vi "test_F9P_ubx-check-2.vi"() -> ()   [LabVIEW 2019]
uses:
  Ctrl/gnss_config.ctl
  Ctrl/ubx-packet.ctl
panel:
  in  "add str":bool=TRUE
  out "ubx arr":T1[](array[typedef])
  in  "GNSS cfg":T2={"Port"="COM10", "heading select"="", "PwrPak7_mode select"=[], "rate"=115200}
  out "buff-n":u32(graph)
  out "data check":bool
  out "error out":errorcluster
  out "n":i32
  out "GNGGA_val":bool
  out "LatLong":cluster{dbl, dbl} {"?" format="%.11f"; "?" format="%.12f"}
  in  "graph arr":bool
  out "XY 그래프":cluster{"X":dbl, "Y":dbl}[](graph)
  in  "정지":bool
  out "연결된 문자열":string
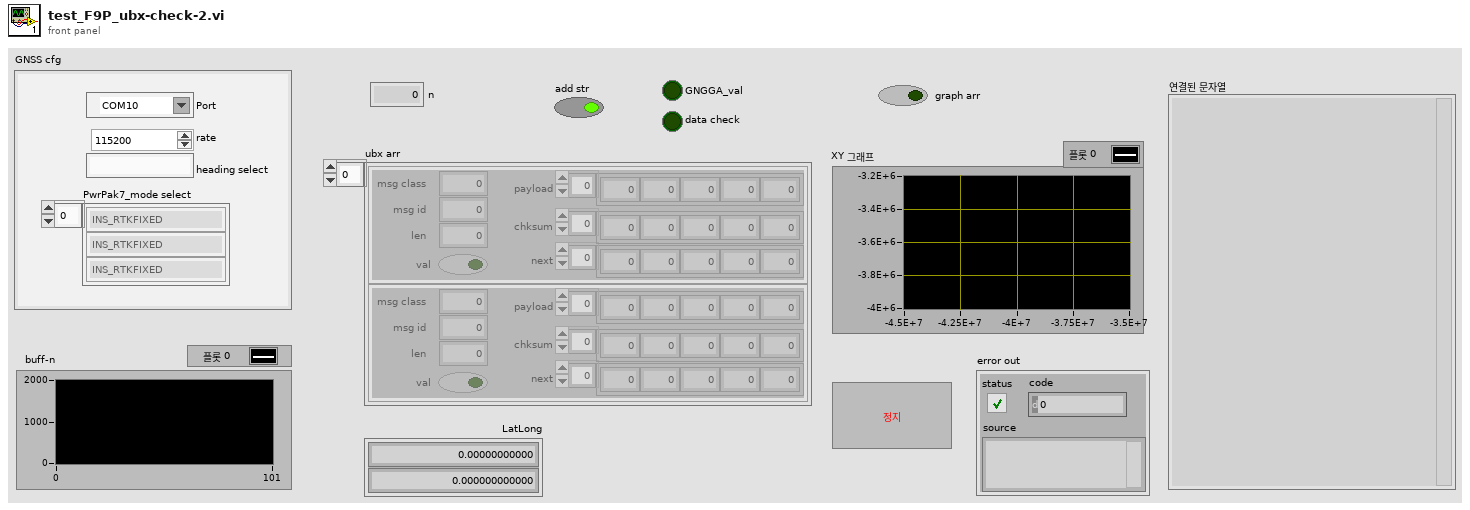
[diagram p1: front panel]
types:
  T1 = typedef "ubx-packet.ctl" = cluster{"msg class":u8, "msg id":u8, "len":u8, "payload":u8[], "chksum":u8[], "next ":u8[], "val":bool}
  T2 = typedef "gnss_config.ctl" = cluster{"Port":refnum<visa-resource-name>, "heading select":string, "PwrPak7_mode select":string[], "rate":u32}
  T3 = enum16{"GxDTM", "GxGBS", "GxGGA", "GxGLL", "GxGNS", "GxGRS", "GxGSA", "GxGST", "GxGSV", "GxRLM", "GxRMC", "GxTHS", "GxTXT", "GxVLW", "GxVTG", "GxZDA"}
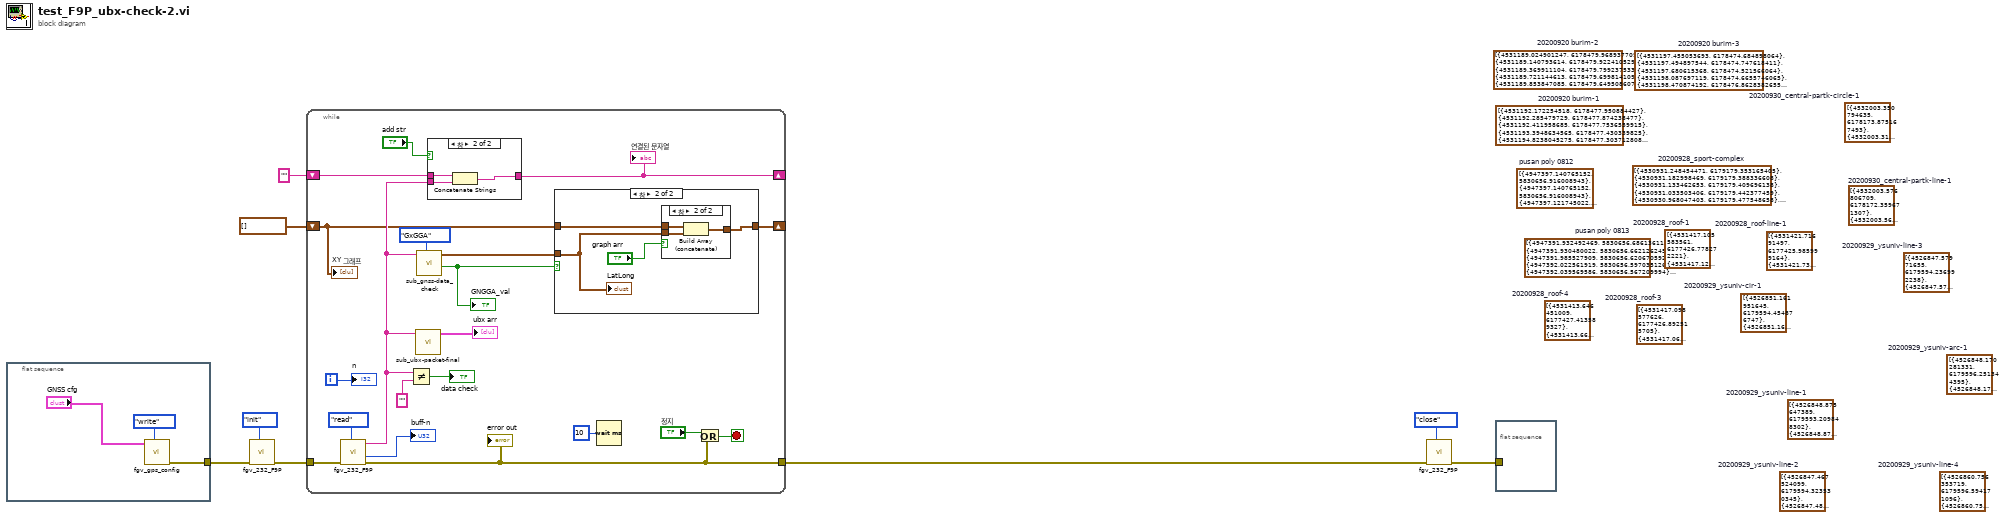
[diagram p0: block diagram]
diagram:
  (unwired) cluster{"X":dbl, "Y":dbl}[] [{"X"=4532003.350794635, "Y"=6178173.875167493}, {"X"=4532003.318056276, "Y"=6178173.892770662}, {"X"=4532003.1579189105, "Y"=6178174.020957441}, {"X"=4532002.967709019, "Y"=6178174.196875582}, {"X"=4532002.672245268, "Y"=6178174.539853451}, {"X"=4532002.3370043775, "Y"=6178175.014684652}, {"X"=4532002.006206528, "Y"=6178175.539729376}, {"X"=4532001.675408691, "Y"=6178176.064773935}, {"X"=4532001.257877701, "Y"=6178176.578591164}, {"X"=4532000.912932229, "Y"=6178177.1375437835}, {"X"=4532000.552950506, "Y"=6178177.72036187}, {"X"=4532000.193857393, "Y"=6178178.313222488}, {"X"=4531999.835652887, "Y"=6178178.916125633}, {"X"=4531999.476559786, "Y"=6178179.508985873}, {"X"=4531998.959036802, "Y"=6178180.055525806}, {"X"=4531998.308713558, "Y"=6178180.457800657}, {"X"=4531997.609657364, "Y"=6178180.696909645}, {"X"=4531996.896383714, "Y"=6178180.775335258}, {"X"=4531996.09371134, "Y"=6178180.812405522}, {"X"=4531995.219342304, "Y"=6178180.814383002}, {"X"=4531994.477703708, "Y"=6178180.766033763}, {"X"=4531993.713031512, "Y"=6178180.651165896}, {"X"=4531992.935100371, "Y"=6178180.580249076}, {"X"=4531992.061620369, "Y"=6178180.592269521}, {"X"=4531991.173992895, "Y"=6178180.638198248}, {"X"=4531990.289920003, "Y"=6178180.724297736}, {"X"=4531989.372220418, "Y"=6178180.817957572}, {"X"=4531988.393487616, "Y"=6178180.997036841}, {"X"=4531987.627109124, "Y"=6178181.056675129}, {"X"=4531986.969538497, "Y"=6178180.989425519}, {"X"=4531986.427884561, "Y"=6178180.875629432}, {"X"=4531985.817199784, "Y"=6178180.75686876}, {"X"=4531985.116227672, "Y"=6178180.586710377}, {"X"=4531984.448882404, "Y"=6178180.408991751}, {"X"=4531983.6541389, "Y"=6178180.341855931}, {"X"=4531982.97797792, "Y"=6178180.258301622}, {"X"=4531982.517725303, "Y"=6178180.095477112}, {"X"=4531982.130876179, "Y"=6178179.793239902}, {"X"=4531982.0643702205, "Y"=6178179.429221983}, {"X"=4531982.268655881, "Y"=6178179.024806436}, {"X"=4531982.716326828, "Y"=6178178.6578521365}, {"X"=4531983.194958756, "Y"=6178178.253209357}, {"X"=4531983.691292785, "Y"=6178177.854828909}, {"X"=4531984.013272379, "Y"=6178177.4239516035}, {"X"=4531984.440575617, "Y"=6178177.020606336}, {"X"=4531984.7652211515, "Y"=6178176.619856802}, {"X"=4531985.021724419, "Y"=6178176.224185293}, {"X"=4531985.4543595435, "Y"=6178175.881095707}, {"X"=4531985.720637784, "Y"=6178175.595893426}, {"X"=4531986.162159305, "Y"=6178175.353230416}, {"X"=4531986.617828416, "Y"=6178175.076659101}, {"X"=4531987.01861415, "Y"=6178174.761214936}, {"X"=4531987.26185866, "Y"=6178174.409493832}, {"X"=4531987.470587696, "Y"=6178174.0552904}, {"X"=4531987.62887644, "Y"=6178173.71242755}, {"X"=4531987.941151956, "Y"=6178173.365670737}, {"X"=4531988.396821304, "Y"=6178173.089098919}, {"X"=4531989.048102098, "Y"=6178172.891456849}, {"X"=4531989.779077613, "Y"=6178172.8192914985}, {"X"=4531990.564048076, "Y"=6178172.775956259}, {"X"=4531991.397681722, "Y"=6178172.701194981}, {"X"=4531992.151691418, "Y"=6178172.6955483295}, {"X"=4531992.878294688, "Y"=6178172.767761083}, {"X"=4531993.734073901, "Y"=6178172.749475895}, {"X"=4531994.601334941, "Y"=6178172.667154285}, {"X"=4531995.4986685645, "Y"=6178172.537101383}, {"X"=4531996.445554117, "Y"=6178172.385665071}, {"X"=4531997.164160308, "Y"=6178172.367493635}, {"X"=4531997.672189098, "Y"=6178172.488849631}, {"X"=4531998.035117029, "Y"=6178172.714526736}, {"X"=4531998.284793752, "Y"=6178173.016879048}, {"X"=4531998.345079205, "Y"=6178173.310600223}, {"X"=4531998.336333534, "Y"=6178173.599356818}, {"X"=4531998.326628996, "Y"=6178173.683478796}, {"X"=4531998.2930020625, "Y"=6178173.691039228}, {"X"=4531998.374403547, "Y"=6178173.642009985}, {"X"=4531999.008942478, "Y"=6178173.642740035}, {"X"=4531999.9470125865, "Y"=6178173.585468922}, {"X"=4532000.815163115, "Y"=6178173.513190527}, {"X"=4532001.679759347, "Y"=6178173.400741216}, {"X"=4532002.4736174755, "Y"=6178173.457834008}, {"X"=4532003.167483395, "Y"=6178173.5476509305}, {"X"=4532003.230364361, "Y"=6178173.67690859}, {"X"=4532003.0135662975, "Y"=6178173.746136882}, {"X"=4532002.899426356, "Y"=6178173.812769338}, {"X"=4532002.781731981, "Y"=6178173.839230853}, {"X"=4532002.700330401, "Y"=6178173.888260139}, {"X"=4532002.602115337, "Y"=6178173.9410696365}, {"X"=4532002.537527241, "Y"=6178173.986318699}, {"X"=4532002.539304456, "Y"=6178174.006404166}, {"X"=4532002.557895154, "Y"=6178174.022709415}, {"X"=4532002.57648585, "Y"=6178174.039014672}, {"X"=4532002.594187939, "Y"=6178174.0452771885}]  # 20200930_central-partk-circle-1
  (unwired) cluster{"X":dbl, "Y":dbl}[] [{"X"=4532003.576806709, "Y"=6178172.359671307}, {"X"=4532003.561770444, "Y"=6178172.383537013}, {"X"=4532003.192762356, "Y"=6178172.4767447}, {"X"=4532002.509629774, "Y"=6178172.702033042}, {"X"=4532001.58140402, "Y"=6178173.064366489}, {"X"=4532000.6080697365, "Y"=6178173.498296774}, {"X"=4531999.621476697, "Y"=6178173.97617793}, {"X"=4531998.631329475, "Y"=6178174.413887931}, {"X"=4531997.607555584, "Y"=6178174.8591581}, {"X"=4531996.653701655, "Y"=6178175.319435316}, {"X"=4531995.644075927, "Y"=6178175.730796639}, {"X"=4531994.618525636, "Y"=6178176.15598064}, {"X"=4531993.592975622, "Y"=6178176.581164397}, {"X"=4531992.5329104, "Y"=6178177.003865606}, {"X"=4531991.489658902, "Y"=6178177.422786382}, {"X"=4531990.527809001, "Y"=6178177.792677899}, {"X"=4531990.226944478, "Y"=6178177.880806713}, {"X"=4531990.291532346, "Y"=6178177.835557892}, {"X"=4531990.903854542, "Y"=6178177.585221218}, {"X"=4531991.817041466, "Y"=6178177.246755574}, {"X"=4531992.795705138, "Y"=6178176.873083589}, {"X"=4531993.754001148, "Y"=6178176.463020804}, {"X"=4531994.714074643, "Y"=6178176.073043199}, {"X"=4531995.743179421, "Y"=6178175.688029997}, {"X"=4531996.772284476, "Y"=6178175.303016582}, {"X"=4531997.801389806, "Y"=6178174.918002955}, {"X"=4531998.829606799, "Y"=6178174.5229464}, {"X"=4531999.824197129, "Y"=6178174.135450053}, {"X"=4532000.801974246, "Y"=6178173.751733712}, {"X"=4532001.763826745, "Y"=6178173.381840121}, {"X"=4532002.707977389, "Y"=6178173.005683826}, {"X"=4532003.204384415, "Y"=6178172.801892536}, {"X"=4532003.252159043, "Y"=6178172.760423654}, {"X"=4532003.199941362, "Y"=6178172.751678849}, {"X"=4532003.165425786, "Y"=6178172.749196558}, {"X"=4532003.130910202, "Y"=6178172.746714265}]  # 20200930_central-partk-line-1
  (unwired) cluster{"X":dbl, "Y":dbl}[] [{"X"=4526860.756353719, "Y"=6179596.594171096}, {"X"=4526860.756353719, "Y"=6179596.594171096}, {"X"=4526860.789939688, "Y"=6179596.586628506}, {"X"=4526860.805839669, "Y"=6179596.572834014}, {"X"=4526860.720981763, "Y"=6179596.581667278}, {"X"=4526860.416922099, "Y"=6179596.629504165}, {"X"=4526859.860967764, "Y"=6179596.733910446}, {"X"=4526859.07080483, "Y"=6179596.901137997}, {"X"=4526858.199356166, "Y"=6179597.1172915315}, {"X"=4526857.262521803, "Y"=6179597.368576525}, {"X"=4526856.323008658, "Y"=6179597.589791859}, {"X"=4526855.407258622, "Y"=6179597.693209538}, {"X"=4526854.471143788, "Y"=6179597.760305785}, {"X"=4526853.586300991, "Y"=6179597.826111375}, {"X"=4526852.740402278, "Y"=6179597.944513448}, {"X"=4526851.791960003, "Y"=6179598.065496877}, {"X"=4526850.8381598815, "Y"=6179598.12634129}, {"X"=4526849.881680892, "Y"=6179598.157116253}, {"X"=4526848.997731885, "Y"=6179598.232945081}, {"X"=4526848.085555225, "Y"=6179598.376455428}, {"X"=4526847.088521079, "Y"=6179598.528798994}, {"X"=4526846.057008274, "Y"=6179598.678661943}, {"X"=4526845.107674283, "Y"=6179598.78962218}, {"X"=4526844.836308457, "Y"=6179598.819893221}, {"X"=4526844.836308457, "Y"=6179598.819893221}, {"X"=4526844.852208359, "Y"=6179598.8060988}]  # 20200929_ysuniv-line-4
  (unwired) cluster{"X":dbl, "Y":dbl}[] [{"X"=4526848.170281331, "Y"=6179596.251344395}, {"X"=4526848.172067365, "Y"=6179596.271390712}, {"X"=4526848.174746415, "Y"=6179596.301460189}, {"X"=4526848.193325387, "Y"=6179596.317735211}, {"X"=4526848.19511142, "Y"=6179596.337781527}, {"X"=4526848.318020094, "Y"=6179596.371521415}, {"X"=4526848.567409516, "Y"=6179596.479093841}, {"X"=4526849.057258204, "Y"=6179596.594007136}, {"X"=4526849.650543608, "Y"=6179596.716362219}, {"X"=4526850.3931795405, "Y"=6179596.784729416}, {"X"=4526851.303745028, "Y"=6179596.815383756}, {"X"=4526852.1675038235, "Y"=6179596.897444746}, {"X"=4526852.889949204, "Y"=6179597.1237023715}, {"X"=4526853.4180231765, "Y"=6179597.475401011}, {"X"=4526853.861239307, "Y"=6179597.835933031}, {"X"=4526854.190476694, "Y"=6179598.262956845}, {"X"=4526854.501135052, "Y"=6179598.673705659}, {"X"=4526854.860386211, "Y"=6179599.053094346}, {"X"=4526855.3195020575, "Y"=6179599.399832276}, {"X"=4526855.828103734, "Y"=6179599.725233304}, {"X"=4526856.067125019, "Y"=6179600.100951621}, {"X"=4526856.206281487, "Y"=6179600.509320781}, {"X"=4526856.273801102, "Y"=6179600.882659113}, {"X"=4526856.14945422, "Y"=6179601.217295914}, {"X"=4526855.675134219, "Y"=6179601.661198722}, {"X"=4526855.062005723, "Y"=6179602.085155568}, {"X"=4526854.368310677, "Y"=6179602.373849684}, {"X"=4526853.501328359, "Y"=6179602.640117238}, {"X"=4526852.607730369, "Y"=6179602.799901114}, {"X"=4526851.800602298, "Y"=6179602.776686818}, {"X"=4526851.081730017, "Y"=6179602.590520808}, {"X"=4526850.492736272, "Y"=6179602.324069063}, {"X"=4526850.067206864, "Y"=6179601.9697890505}, {"X"=4526849.843192611, "Y"=6179601.570253982}, {"X"=4526849.956823016, "Y"=6179601.115339965}, {"X"=4526849.968802758, "Y"=6179600.673030329}, {"X"=4526849.760688252, "Y"=6179600.259700865}, {"X"=4526849.320151586, "Y"=6179599.929238734}, {"X"=4526848.731157484, "Y"=6179599.662787635}, {"X"=4526848.168779378, "Y"=6179599.502820084}, {"X"=4526847.817739581, "Y"=6179599.407851984}, {"X"=4526847.179433946, "Y"=6179599.356949316}, {"X"=4526846.581684026, "Y"=6179599.184478212}, {"X"=4526846.227790916, "Y"=6179598.865229688}, {"X"=4526846.242449157, "Y"=6179598.452989891}, {"X"=4526846.59921707, "Y"=6179598.035486411}, {"X"=4526847.123021329, "Y"=6179597.570246789}, {"X"=4526847.458531307, "Y"=6179597.106398559}, {"X"=4526847.916056945, "Y"=6179596.666266938}, {"X"=4526848.549549199, "Y"=6179596.27863064}, {"X"=4526849.392594041, "Y"=6179595.935947071}, {"X"=4526850.155420726, "Y"=6179595.846423975}, {"X"=4526850.457693785, "Y"=6179595.778540601}, {"X"=4526850.523079555, "Y"=6179595.743409067}, {"X"=4526850.637058142, "Y"=6179595.676917302}, {"X"=4526850.734243783, "Y"=6179595.614196826}, {"X"=4526850.832322437, "Y"=6179595.561499524}, {"X"=4526850.895922179, "Y"=6179595.506321643}]  # 20200929_ysuniv-arc-1
  (unwired) cluster{"X":dbl, "Y":dbl}[] [{"X"=4526847.57971655, "Y"=6179594.236992238}, {"X"=4526847.578823527, "Y"=6179594.226969077}, {"X"=4526847.5779305035, "Y"=6179594.216945917}, {"X"=4526847.577037481, "Y"=6179594.206922759}, {"X"=4526847.817496807, "Y"=6179594.214263396}, {"X"=4526848.30377362, "Y"=6179594.28908366}, {"X"=4526848.877587275, "Y"=6179594.385140075}, {"X"=4526849.469979942, "Y"=6179594.49747158}, {"X"=4526850.149909467, "Y"=6179594.6310392935}, {"X"=4526850.917375851, "Y"=6179594.785843256}, {"X"=4526851.720214229, "Y"=6179594.953151071}, {"X"=4526852.541631642, "Y"=6179595.136734074}, {"X"=4526853.345363136, "Y"=6179595.314065338}, {"X"=4526854.151773704, "Y"=6179595.5214662915}, {"X"=4526854.942284363, "Y"=6179595.7426618785}, {"X"=4526855.729223025, "Y"=6179595.923764881}, {"X"=4526856.532061694, "Y"=6179596.091073533}, {"X"=4526857.301314478, "Y"=6179596.265924913}, {"X"=4526858.087360279, "Y"=6179596.437005135}, {"X"=4526858.874299126, "Y"=6179596.61810868}, {"X"=4526859.578166127, "Y"=6179596.828092018}, {"X"=4526860.330626089, "Y"=6179597.006715212}, {"X"=4526861.154722999, "Y"=6179597.22036939}, {"X"=4526861.497007489, "Y"=6179597.409318161}, {"X"=4526861.4528794885, "Y"=6179597.490794452}, {"X"=4526861.303528628, "Y"=6179597.544782445}, {"X"=4526861.2054497115, "Y"=6179597.597479778}, {"X"=4526861.072891846, "Y"=6179597.647696484}]  # 20200929_ysuniv-line-3
  (unwired) cluster{"X":dbl, "Y":dbl}[] [{"X"=4526847.467524099, "Y"=6179594.323530345}, {"X"=4526847.485210063, "Y"=6179594.329782201}, {"X"=4526847.502896027, "Y"=6179594.336034054}, {"X"=4526847.571853841, "Y"=6179594.340995139}, {"X"=4526847.697441634, "Y"=6179594.40480442}, {"X"=4526847.892880264, "Y"=6179594.483597957}, {"X"=4526848.236776315, "Y"=6179594.498380264}, {"X"=4526848.501172765, "Y"=6179594.582134931}, {"X"=4526848.667490617, "Y"=6179594.718586936}, {"X"=4526848.802901622, "Y"=6179594.892651054}, {"X"=4526848.939205637, "Y"=6179595.0767383445}, {"X"=4526849.057823673, "Y"=6179595.254573792}, {"X"=4526849.177334716, "Y"=6179595.442432413}, {"X"=4526849.329538613, "Y"=6179595.612725276}, {"X"=4526849.498535446, "Y"=6179595.779246859}, {"X"=4526849.732025003, "Y"=6179595.900613774}, {"X"=4526849.999100443, "Y"=6179596.014438112}, {"X"=4526850.33066864, "Y"=6179596.083107786}, {"X"=4526850.781573511, "Y"=6179596.145424739}, {"X"=4526851.3350221235, "Y"=6179596.2051602965}, {"X"=4526851.972435541, "Y"=6179596.246039417}, {"X"=4526852.642541916, "Y"=6179596.269352819}, {"X"=4526853.4125131, "Y"=6179596.260015311}, {"X"=4526854.168370443, "Y"=6179596.284518674}, {"X"=4526854.859735047, "Y"=6179596.354176823}, {"X"=4526855.454806941, "Y"=6179596.496578729}, {"X"=4526855.918214148, "Y"=6179596.699220611}, {"X"=4526856.253528623, "Y"=6179597.002195207}, {"X"=4526856.42269941, "Y"=6179597.36292913}, {"X"=4526856.44341244, "Y"=6179597.787674212}, {"X"=4526856.4171445295, "Y"=6179598.069614061}, {"X"=4526856.4412554875, "Y"=6179598.340240047}, {"X"=4526856.641333033, "Y"=6179598.66336188}, {"X"=4526857.121532972, "Y"=6179598.862232873}, {"X"=4526857.633532847, "Y"=6179599.0335150175}, {"X"=4526857.742327595, "Y"=6179599.101096036}, {"X"=4526857.677834711, "Y"=6179599.146250714}, {"X"=4526857.629241795, "Y"=6179599.177610924}, {"X"=4526857.581541879, "Y"=6179599.218994313}, {"X"=4526857.549741936, "Y"=6179599.246583243}, {"X"=4526857.500256033, "Y"=6179599.267920262}]  # 20200929_ysuniv-line-2
  (unwired) cluster{"X":dbl, "Y":dbl}[] [{"X"=4526848.875647389, "Y"=6179593.209848302}, {"X"=4526848.878326462, "Y"=6179593.239917798}, {"X"=4526848.898691504, "Y"=6179593.276239142}, {"X"=4526849.058758274, "Y"=6179593.342528971}, {"X"=4526849.445170584, "Y"=6179593.450000222}, {"X"=4526849.882854773, "Y"=6179593.556180745}, {"X"=4526850.441661731, "Y"=6179593.676054804}, {"X"=4526851.08443348, "Y"=6179593.777072374}, {"X"=4526851.7943771025, "Y"=6179593.863004775}, {"X"=4526852.537906699, "Y"=6179593.941394629}, {"X"=4526853.28232938, "Y"=6179594.02980775}, {"X"=4526854.001203319, "Y"=6179594.215972202}, {"X"=4526854.606098577, "Y"=6179594.468628661}, {"X"=4526855.01305027, "Y"=6179594.806633645}, {"X"=4526855.533980649, "Y"=6179595.07814685}, {"X"=4526856.187468742, "Y"=6179595.299443374}, {"X"=4526856.939928663, "Y"=6179595.478065833}, {"X"=4526857.7391955275, "Y"=6179595.605281743}, {"X"=4526857.952320257, "Y"=6179595.690327663}, {"X"=4526858.317474763, "Y"=6179595.7514550835}, {"X"=4526858.855917065, "Y"=6179595.835008726}, {"X"=4526859.448310326, "Y"=6179595.947341314}, {"X"=4526859.94173174, "Y"=6179596.102348155}, {"X"=4526860.47231111, "Y"=6179596.2899052715}, {"X"=4526861.089534393, "Y"=6179596.488675603}, {"X"=4526861.743915627, "Y"=6179596.719996271}, {"X"=4526862.364710898, "Y"=6179596.958859657}, {"X"=4526862.492977711, "Y"=6179597.052739102}, {"X"=4526862.461177725, "Y"=6179597.080328097}, {"X"=4526862.410798762, "Y"=6179597.091641968}, {"X"=4526862.343626815, "Y"=6179597.106727131}]  # 20200929_ysuniv-line-1
  (unwired) cluster{"X":dbl, "Y":dbl}[] [{"X"=4526851.161951645, "Y"=6179594.454876747}, {"X"=4526851.160165612, "Y"=6179594.434830405}, {"X"=4526851.158379577, "Y"=6179594.414784061}, {"X"=4526851.663061232, "Y"=6179594.311667998}, {"X"=4526852.482518404, "Y"=6179594.2809928255}, {"X"=4526853.345384775, "Y"=6179594.353030039}, {"X"=4526854.162337407, "Y"=6179594.486497184}, {"X"=4526855.026096969, "Y"=6179594.568557794}, {"X"=4526855.826256791, "Y"=6179594.705796473}, {"X"=4526856.5574587695, "Y"=6179594.838074114}, {"X"=4526857.139310055, "Y"=6179595.024339973}, {"X"=4526857.654882454, "Y"=6179595.235714333}, {"X"=4526858.115610911, "Y"=6179595.408286708}, {"X"=4526858.6461902745, "Y"=6179595.595843531}, {"X"=4526859.013304869, "Y"=6179595.871229412}, {"X"=4526859.1710407045, "Y"=6179596.2958741775}, {"X"=4526858.990237959, "Y"=6179596.765875233}, {"X"=4526858.400152833, "Y"=6179597.256224802}, {"X"=4526857.777374863, "Y"=6179597.764139932}, {"X"=4526857.309305699, "Y"=6179598.27820603}, {"X"=4526856.946459353, "Y"=6179598.819760186}, {"X"=4526856.493397248, "Y"=6179599.310008271}, {"X"=4526855.849361673, "Y"=6179599.771577935}, {"X"=4526855.018817709, "Y"=6179600.254585023}, {"X"=4526854.047679364, "Y"=6179600.697599781}, {"X"=4526853.097625223, "Y"=6179600.992747389}, {"X"=4526852.132390359, "Y"=6179601.117501036}, {"X"=4526851.191811576, "Y"=6179601.134480512}, {"X"=4526850.343060566, "Y"=6179601.028600849}, {"X"=4526849.622402106, "Y"=6179600.822389063}, {"X"=4526849.063421987, "Y"=6179600.508302624}, {"X"=4526848.455849041, "Y"=6179600.225576438}, {"X"=4526847.704283764, "Y"=6179600.056977049}, {"X"=4526846.82105413, "Y"=6179599.948617422}, {"X"=4526845.83885306, "Y"=6179599.882931848}, {"X"=4526844.939723721, "Y"=6179599.788366873}, {"X"=4526844.370201775, "Y"=6179599.548214539}, {"X"=4526844.012736666, "Y"=6179599.188873723}, {"X"=4526843.85589351, "Y"=6179598.774254482}, {"X"=4526843.950944102, "Y"=6179598.303066019}, {"X"=4526844.216602938, "Y"=6179597.824234059}, {"X"=4526844.601598294, "Y"=6179597.339049252}, {"X"=4526844.940679999, "Y"=6179596.915293892}, {"X"=4526845.4839559365, "Y"=6179596.476352336}, {"X"=4526846.0626038695, "Y"=6179596.049914321}, {"X"=4526846.94888287, "Y"=6179595.615731669}, {"X"=4526847.891792053, "Y"=6179595.240396991}, {"X"=4526848.876324531, "Y"=6179594.947727983}, {"X"=4526849.243090278, "Y"=6179594.8346897885}, {"X"=4526849.342954935, "Y"=6179594.802038793}, {"X"=4526849.444605636, "Y"=6179594.789434132}, {"X"=4526849.527677354, "Y"=6179594.760554434}, {"X"=4526849.611642092, "Y"=6179594.741697908}, {"X"=4526850.21440221, "Y"=6179594.5858845655}, {"X"=4526850.568840211, "Y"=6179594.5267334655}, {"X"=4526850.653697985, "Y"=6179594.517900102}, {"X"=4526850.738555764, "Y"=6179594.509066738}, {"X"=4526850.80572757, "Y"=6179594.493981508}, {"X"=4526850.890585347, "Y"=6179594.485148147}, {"X"=4526850.941857225, "Y"=6179594.483857392}]  # 20200929_ysuniv-cir-1
  (unwired) cluster{"X":dbl, "Y":dbl}[] [{"X"=4531421.71691497, "Y"=6177425.985999164}, {"X"=4531421.733727922, "Y"=6177425.982214279}, {"X"=4531421.768245372, "Y"=6177425.984686208}, {"X"=4531421.785949871, "Y"=6177425.990943029}, {"X"=4531421.671825347, "Y"=6177426.057604076}, {"X"=4531421.4046011595, "Y"=6177426.138245689}, {"X"=4531421.0878296755, "Y"=6177426.240283662}, {"X"=4531420.686993459, "Y"=6177426.361246052}, {"X"=4531420.351625991, "Y"=6177426.446985468}, {"X"=4531419.965819711, "Y"=6177426.544079531}, {"X"=4531419.511870139, "Y"=6177426.646271414}, {"X"=4531419.025186271, "Y"=6177426.766074745}, {"X"=4531418.522581059, "Y"=6177426.899704632}, {"X"=4531417.998705244, "Y"=6177426.986910897}, {"X"=4531416.675706004, "Y"=6177427.151589676}, {"X"=4531416.166860236, "Y"=6177427.214927659}, {"X"=4531415.675719008, "Y"=6177427.284522443}, {"X"=4531415.218203677, "Y"=6177427.346547468}, {"X"=4531414.282794047, "Y"=6177427.434215655}, {"X"=4531413.957999157, "Y"=6177427.445878289}, {"X"=4531413.788086804, "Y"=6177427.463643719}, {"X"=4531413.600469985, "Y"=6177427.475152356}, {"X"=4531413.189827422, "Y"=6177427.485656033}, {"X"=4531412.663277538, "Y"=6177427.542737218}, {"X"=4531412.108451183, "Y"=6177427.667638201}, {"X"=4531411.583684528, "Y"=6177427.744802721}, {"X"=4531411.092543752, "Y"=6177427.8143974785}, {"X"=4531410.635028868, "Y"=6177427.876422473}, {"X"=4531410.193435373, "Y"=6177427.924620927}, {"X"=4531409.7509503625, "Y"=6177427.962777718}, {"X"=4531409.376608583, "Y"=6177427.995836669}, {"X"=4531409.035001097, "Y"=6177428.011284209}, {"X"=4531407.384535112, "Y"=6177428.1575006135}, {"X"=4531406.48364428, "Y"=6177428.247640767}, {"X"=4531405.941173767, "Y"=6177428.318548476}, {"X"=4531405.7331781015, "Y"=6177428.293675412}]  # 20200928_roof-line-1
  (unwired) cluster{"X":dbl, "Y":dbl}[] [{"X"=4531413.646451009, "Y"=6177427.413589327}, {"X"=4531413.663263937, "Y"=6177427.40980445}, {"X"=4531413.663263937, "Y"=6177427.40980445}, {"X"=4531413.64555946, "Y"=6177427.403547649}, {"X"=4531413.6446679095, "Y"=6177427.393505972}, {"X"=4531413.6446679095, "Y"=6177427.393505972}, {"X"=4531413.6446679095, "Y"=6177427.393505972}, {"X"=4531413.64377636, "Y"=6177427.383464294}, {"X"=4531413.454376446, "Y"=6177427.374889576}, {"X"=4531412.872038456, "Y"=6177427.383075364}, {"X"=4531412.033048975, "Y"=6177427.397826003}, {"X"=4531411.133048829, "Y"=6177427.498007888}, {"X"=4531410.204772342, "Y"=6177427.666009528}, {"X"=4531409.192431507, "Y"=6177427.852935506}, {"X"=4531408.129652185, "Y"=6177428.051216055}, {"X"=4531407.081902899, "Y"=6177428.225628358}, {"X"=4531406.276540151, "Y"=6177428.232809343}, {"X"=4531405.610903278, "Y"=6177428.075385062}, {"X"=4531405.054932643, "Y"=6177427.801091911}, {"X"=4531404.562647289, "Y"=6177427.47149278}, {"X"=4531404.307525526, "Y"=6177427.108988701}, {"X"=4531404.170985528, "Y"=6177426.73003214}, {"X"=4531404.198116579, "Y"=6177426.263018489}, {"X"=4531404.443815216, "Y"=6177425.746801235}, {"X"=4531404.8647753885, "Y"=6177425.273068127}, {"X"=4531405.481376355, "Y"=6177424.878200854}, {"X"=4531406.224583443, "Y"=6177424.5572557}, {"X"=4531407.161648367, "Y"=6177424.295093113}, {"X"=4531408.203157243, "Y"=6177424.050387671}, {"X"=4531409.268611818, "Y"=6177423.882230574}, {"X"=4531410.241213201, "Y"=6177423.827157895}, {"X"=4531411.183755164, "Y"=6177423.819821749}, {"X"=4531412.082099425, "Y"=6177423.894132112}, {"X"=4531412.849506615, "Y"=6177424.03888851}, {"X"=4531413.485085084, "Y"=6177424.244049259}, {"X"=4531413.887957195, "Y"=6177424.532323746}, {"X"=4531413.957245314, "Y"=6177424.926421259}, {"X"=4531413.656648938, "Y"=6177425.403786396}, {"X"=4531413.170218833, "Y"=6177425.912743506}, {"X"=4531412.58201969, "Y"=6177426.434368061}, {"X"=4531411.886702254, "Y"=6177426.908409978}, {"X"=4531411.433771617, "Y"=6177427.215220101}, {"X"=4531411.354164798, "Y"=6177427.284352858}, {"X"=4531411.371869269, "Y"=6177427.290609647}, {"X"=4531411.389573738, "Y"=6177427.296866437}, {"X"=4531411.406386656, "Y"=6177427.293081557}, {"X"=4531411.440904046, "Y"=6177427.295553469}, {"X"=4531411.458608513, "Y"=6177427.301810261}, {"X"=4531411.493125904, "Y"=6177427.304282171}, {"X"=4531411.509938822, "Y"=6177427.300497289}, {"X"=4531411.526751735, "Y"=6177427.296712409}]  # 20200928_roof-4
  (unwired) cluster{"X":dbl, "Y":dbl}[] [{"X"=4531417.098577626, "Y"=6177426.892515705}, {"X"=4531417.063168656, "Y"=6177426.880002091}, {"X"=4531417.010946754, "Y"=6177426.871273357}, {"X"=4531416.975537794, "Y"=6177426.858759739}, {"X"=4531416.940128824, "Y"=6177426.84624613}, {"X"=4531416.836576568, "Y"=6177426.838830355}, {"X"=4531416.663989472, "Y"=6177426.826470736}, {"X"=4531416.458668056, "Y"=6177426.831722575}, {"X"=4531416.114385437, "Y"=6177426.817045048}, {"X"=4531415.756856092, "Y"=6177426.846319155}, {"X"=4531415.262148679, "Y"=6177426.875747278}, {"X"=4531414.612558748, "Y"=6177426.899072617}, {"X"=4531413.790381877, "Y"=6177426.910038413}, {"X"=4531412.873568446, "Y"=6177427.01400527}, {"X"=4531411.960321403, "Y"=6177427.1581388265}, {"X"=4531411.0152318105, "Y"=6177427.329925446}, {"X"=4531410.04798017, "Y"=6177427.445246913}, {"X"=4531409.05156069, "Y"=6177427.61834643}, {"X"=4531408.01794939, "Y"=6177427.758849023}, {"X"=4531406.951604062, "Y"=6177427.916963009}, {"X"=4531405.981678558, "Y"=6177428.002159455}, {"X"=4531405.1523705395, "Y"=6177427.932792254}, {"X"=4531404.705301322, "Y"=6177427.726164743}, {"X"=4531404.536918758, "Y"=6177427.374861184}, {"X"=4531404.5348819485, "Y"=6177426.965625536}, {"X"=4531404.66913139, "Y"=6177426.546194078}, {"X"=4531405.075953437, "Y"=6177426.106370957}, {"X"=4531405.759806033, "Y"=6177425.696364327}, {"X"=4531406.613570934, "Y"=6177425.268591908}, {"X"=4531407.513443779, "Y"=6177424.973832717}, {"X"=4531408.508971739, "Y"=6177424.790690551}, {"X"=4531409.5965885725, "Y"=6177424.678998852}, {"X"=4531410.62141177, "Y"=6177424.63265511}, {"X"=4531411.581658146, "Y"=6177424.63157602}, {"X"=4531412.464972509, "Y"=6177424.729754914}, {"X"=4531413.250084078, "Y"=6177424.880768327}, {"X"=4531414.020165881, "Y"=6177425.05565013}, {"X"=4531414.691153239, "Y"=6177425.273324783}, {"X"=4531415.2825337015, "Y"=6177425.560132456}, {"X"=4531415.826149982, "Y"=6177425.888419979}, {"X"=4531416.09006067, "Y"=6177426.1567655625}, {"X"=4531416.200745323, "Y"=6177426.244514813}, {"X"=4531416.241503579, "Y"=6177426.317278551}, {"X"=4531416.284936479, "Y"=6177426.420167352}, {"X"=4531416.400078862, "Y"=6177426.558125059}, {"X"=4531416.46478243, "Y"=6177426.707437428}, {"X"=4531416.548973554, "Y"=6177426.883089987}, {"X"=4531416.502100938, "Y"=6177426.934611387}, {"X"=4531416.449879036, "Y"=6177426.925882657}, {"X"=4531416.379952658, "Y"=6177426.910897125}, {"X"=4531416.3268392095, "Y"=6177426.892126706}, {"X"=4531416.256912837, "Y"=6177426.87714117}]  # 20200928_roof-3
  (unwired) cluster{"X":dbl, "Y":dbl}[] [{"X"=4531417.105583561, "Y"=6177426.778272221}, {"X"=4531417.122396494, "Y"=6177426.774487338}, {"X"=4531417.122396494, "Y"=6177426.774487338}, {"X"=4531417.071066141, "Y"=6177426.775800299}, {"X"=4531416.6162253, "Y"=6177426.867950453}, {"X"=4531416.109162615, "Y"=6177426.951371864}, {"X"=4531415.599425339, "Y"=6177427.0046682125}, {"X"=4531415.001165723, "Y"=6177427.026680552}, {"X"=4531414.43296583, "Y"=6177427.000956415}, {"X"=4531413.950613719, "Y"=6177426.976391261}, {"X"=4531413.36560099, "Y"=6177426.954452078}, {"X"=4531412.660223198, "Y"=6177426.928882076}, {"X"=4531412.170738786, "Y"=6177426.823983625}, {"X"=4531411.812191528, "Y"=6177426.648639461}, {"X"=4531411.688133576, "Y"=6177426.41026528}, {"X"=4531411.756023529, "Y"=6177426.01601405}, {"X"=4531411.891165139, "Y"=6177425.606623218}, {"X"=4531412.09444998, "Y"=6177425.192134425}, {"X"=4531412.384474118, "Y"=6177424.788846096}, {"X"=4531412.848868456, "Y"=6177424.418000451}, {"X"=4531413.439868958, "Y"=6177424.121077197}, {"X"=4531414.124741367, "Y"=6177423.9156878535}, {"X"=4531414.902594141, "Y"=6177423.791790808}, {"X"=4531415.625677085, "Y"=6177423.823617006}, {"X"=4531416.155920366, "Y"=6177424.001278992}, {"X"=4531416.592418442, "Y"=6177424.281983991}, {"X"=4531416.9147921, "Y"=6177424.62935013}, {"X"=4531417.138071152, "Y"=6177425.019509088}, {"X"=4531417.244551113, "Y"=6177425.446204018}, {"X"=4531417.2837792495, "Y"=6177425.888038506}, {"X"=4531417.153986394, "Y"=6177426.357680148}, {"X"=4531416.9551586695, "Y"=6177426.8223778615}, {"X"=4531416.851732848, "Y"=6177427.009539084}, {"X"=4531416.819890063, "Y"=6177427.037192224}, {"X"=4531416.80218558, "Y"=6177427.030935412}, {"X"=4531416.767668164, "Y"=6177427.028463492}, {"X"=4531416.750855228, "Y"=6177427.03224837}, {"X"=4531416.716337811, "Y"=6177427.029776447}]  # 20200928_roof-1
  (unwired) cluster{"X":dbl, "Y":dbl}[] [{"X"=4530931.248454471, "Y"=6179179.353165405}, {"X"=4530931.182998469, "Y"=6179179.388336608}, {"X"=4530931.133462653, "Y"=6179179.409696138}, {"X"=4530931.033503406, "Y"=6179179.442377459}, {"X"=4530930.968047403, "Y"=6179179.477548658}, {"X"=4530931.267925158, "Y"=6179179.379504706}, {"X"=4530932.021613948, "Y"=6179179.179564613}, {"X"=4530932.9433810655, "Y"=6179178.941885138}, {"X"=4530933.95362562, "Y"=6179178.735524664}, {"X"=4530934.990442061, "Y"=6179178.635805512}, {"X"=4530935.978610454, "Y"=6179178.567483689}, {"X"=4530936.761591465, "Y"=6179178.698789498}, {"X"=4530937.213741527, "Y"=6179178.965800651}, {"X"=4530937.551787178, "Y"=6179179.299380458}, {"X"=4530937.787210536, "Y"=6179179.635528379}, {"X"=4530937.8890587855, "Y"=6179180.011905499}, {"X"=4530937.825491477, "Y"=6179180.456135154}, {"X"=4530937.590295369, "Y"=6179180.897952905}, {"X"=4530937.110913539, "Y"=6179181.292227798}, {"X"=4530936.476710887, "Y"=6179181.680316756}, {"X"=4530935.682361836, "Y"=6179182.001993222}, {"X"=4530934.81545601, "Y"=6179182.278538684}, {"X"=4530933.939674247, "Y"=6179182.454706554}, {"X"=4530933.023176129, "Y"=6179182.558120229}, {"X"=4530932.121710757, "Y"=6179182.637684509}, {"X"=4530931.28570154, "Y"=6179182.682077687}, {"X"=4530930.386899324, "Y"=6179182.7917552125}, {"X"=4530929.454481665, "Y"=6179182.908980536}, {"X"=4530928.61231651, "Y"=6179183.077600423}, {"X"=4530927.720615753, "Y"=6179183.267579702}, {"X"=4530926.826252312, "Y"=6179183.427445762}, {"X"=4530925.896498235, "Y"=6179183.574784142}, {"X"=4530925.0162800625, "Y"=6179183.700763071}, {"X"=4530924.133399187, "Y"=6179183.796628841}, {"X"=4530923.250518463, "Y"=6179183.892494618}, {"X"=4530922.421611728, "Y"=6179184.017189509}, {"X"=4530921.57767262, "Y"=6179184.165733692}, {"X"=4530920.92832585, "Y"=6179184.18868945}, {"X"=4530920.467357915, "Y"=6179184.015792938}, {"X"=4530920.2655503, "Y"=6179183.672099369}, {"X"=4530920.319409679, "Y"=6179183.311948054}, {"X"=4530920.648406759, "Y"=6179182.961678103}, {"X"=4530921.254316909, "Y"=6179182.641364853}, {"X"=4530922.079615876, "Y"=6179182.282028339}, {"X"=4530922.994279711, "Y"=6179181.964048354}, {"X"=4530923.919595313, "Y"=6179181.7665208}, {"X"=4530924.876751438, "Y"=6179181.541369912}, {"X"=4530925.755194588, "Y"=6179181.395314856}, {"X"=4530926.596471808, "Y"=6179181.216656706}, {"X"=4530927.467814283, "Y"=6179180.990299754}, {"X"=4530928.302878458, "Y"=6179180.7413773695}, {"X"=4530929.087519394, "Y"=6179180.503776652}, {"X"=4530929.9526490215, "Y"=6179180.2071552705}, {"X"=4530930.201215633, "Y"=6179180.110395453}, {"X"=4530930.216248196, "Y"=6179180.08654605}, {"X"=4530930.611646993, "Y"=6179179.905632181}, {"X"=4530930.759366785, "Y"=6179179.831515882}, {"X"=4530930.743446603, "Y"=6179179.845327551}, {"X"=4530930.726638794, "Y"=6179179.849101472}, {"X"=4530930.70716811, "Y"=6179179.82276218}, {"X"=4530930.721313046, "Y"=6179179.7888750285}, {"X"=4530930.702729987, "Y"=6179179.772573478}, {"X"=4530930.913242909, "Y"=6179179.633172752}, {"X"=4530931.516491869, "Y"=6179179.28274478}, {"X"=4530931.711084643, "Y"=6179179.157155663}, {"X"=4530932.136548748, "Y"=6179178.928542747}, {"X"=4530932.261247414, "Y"=6179178.787936073}, {"X"=4530932.293975424, "Y"=6179178.770350455}, {"X"=4530932.342623632, "Y"=6179178.738953164}, {"X"=4530932.424887473, "Y"=6179178.700008001}, {"X"=4530932.373576393, "Y"=6179178.701292055}, {"X"=4530932.371801144, "Y"=6179178.681216558}, {"X"=4530932.372688769, "Y"=6179178.691254306}, {"X"=4530932.373576393, "Y"=6179178.701292055}]  # 20200928_sport-complex
  (unwired) cluster{"X":dbl, "Y":dbl}[] [{"X"=4531197.455053693, "Y"=6178474.684898064}, {"X"=4531197.494897544, "Y"=6178474.747618411}, {"X"=4531197.680615368, "Y"=6178474.521566064}, {"X"=4531198.087697119, "Y"=6178474.6655746065}, {"X"=4531198.470874192, "Y"=6178476.8628382655}, {"X"=4531199.832329028, "Y"=6178476.167733575}, {"X"=4531202.209422474, "Y"=6178475.131714717}, {"X"=4531202.904943879, "Y"=6178475.241610843}, {"X"=4531205.717736307, "Y"=6178475.059928495}, {"X"=4531206.237154929, "Y"=6178475.117251794}, {"X"=4531207.058267196, "Y"=6178475.096525569}, {"X"=4531208.554535095, "Y"=6178475.149315897}, {"X"=4531210.150857343, "Y"=6178475.363927885}, {"X"=4531211.771020513, "Y"=6178475.460547793}, {"X"=4531212.589466312, "Y"=6178475.4097030945}, {"X"=4531212.874350115, "Y"=6178475.335431868}, {"X"=4531216.452168476, "Y"=6178474.305996676}, {"X"=4531216.395596452, "Y"=6178474.441585692}, {"X"=4531216.50704432, "Y"=6178474.344859869}, {"X"=4531216.958170187, "Y"=6178474.018194333}, {"X"=4531216.68128763, "Y"=6178474.182822483}, {"X"=4531216.660032155, "Y"=6178474.136402619}, {"X"=4531216.605156303, "Y"=6178474.097539429}, {"X"=4531216.543167978, "Y"=6178473.978359118}, {"X"=4531216.562563386, "Y"=6178473.810168191}, {"X"=4531216.4590351, "Y"=6178473.802719311}, {"X"=4531216.4306671275, "Y"=6178473.675982325}, {"X"=4531218.525061565, "Y"=6178471.577158608}, {"X"=4531219.621759752, "Y"=6178470.409104861}, {"X"=4531220.302812468, "Y"=6178469.774771379}, {"X"=4531221.946082463, "Y"=6178468.002608739}, {"X"=4531222.196293424, "Y"=6178467.536789631}, {"X"=4531222.481902952, "Y"=6178467.083492994}, {"X"=4531222.595936115, "Y"=6178466.822353526}, {"X"=4531222.755954585, "Y"=6178466.499680512}, {"X"=4531223.047705491, "Y"=6178465.92212916}, {"X"=4531223.213058378, "Y"=6178465.659694057}, {"X"=4531223.553461806, "Y"=6178465.050727936}, {"X"=4531223.57196802, "Y"=6178464.872496655}, {"X"=4531223.930070735, "Y"=6178464.269791578}, {"X"=4531224.240492173, "Y"=6178463.903072883}, {"X"=4531224.588008209, "Y"=6178463.374423658}, {"X"=4531225.072673359, "Y"=6178462.845666068}, {"X"=4531225.271646757, "Y"=6178462.575673688}, {"X"=4531225.486541321, "Y"=6178462.291863172}, {"X"=4531225.653672402, "Y"=6178462.049506905}, {"X"=4531226.54428626, "Y"=6178461.071120812}, {"X"=4531226.775102048, "Y"=6178460.773491903}, {"X"=4531227.1527646715, "Y"=6178460.391658659}, {"X"=4531228.075945708, "Y"=6178459.0066094315}, {"X"=4531228.204121863, "Y"=6178458.711571338}, {"X"=4531228.397760873, "Y"=6178458.381340067}, {"X"=4531228.955808738, "Y"=6178457.713212052}, {"X"=4531229.191070042, "Y"=6178457.465781055}, {"X"=4531229.5739850355, "Y"=6178456.949652315}, {"X"=4531229.724305976, "Y"=6178456.711073706}, {"X"=4531229.906469266, "Y"=6178456.444858751}, {"X"=4531230.076185366, "Y"=6178456.038087816}, {"X"=4531230.107056261, "Y"=6178455.805878833}, {"X"=4531230.003445011, "Y"=6178455.603897468}, {"X"=4531229.913976741, "Y"=6178455.368018527}, {"X"=4531229.778523102, "Y"=6178455.1936735}, {"X"=4531229.48119041, "Y"=6178455.127391025}, {"X"=4531229.152904471, "Y"=6178455.098784606}, {"X"=4531228.819283991, "Y"=6178455.009939962}, {"X"=4531227.802666452, "Y"=6178455.14629}, {"X"=4531227.31250166, "Y"=6178455.225746112}, {"X"=4531226.8355907975, "Y"=6178455.261264957}, {"X"=4531226.457763322, "Y"=6178455.254033679}, {"X"=4531224.9306150805, "Y"=6178455.433459477}, {"X"=4531224.27056991, "Y"=6178455.530620715}, {"X"=4531223.506189583, "Y"=6178455.804826439}, {"X"=4531222.012745413, "Y"=6178456.1712276125}, {"X"=4531221.352700678, "Y"=6178456.2683887305}, {"X"=4531220.7262765, "Y"=6178456.357992939}, {"X"=4531220.101630612, "Y"=6178456.467676488}, {"X"=4531218.390461072, "Y"=6178456.698704554}, {"X"=4531217.810911532, "Y"=6178456.736814711}, {"X"=4531212.991383478, "Y"=6178457.103338522}, {"X"=4531212.380881459, "Y"=6178457.179124597}, {"X"=4531211.24651304, "Y"=6178457.147391773}, {"X"=4531210.620979255, "Y"=6178457.247035602}, {"X"=4531209.926426552, "Y"=6178457.3417139035}, {"X"=4531208.262774573, "Y"=6178456.947693293}, {"X"=4531207.77608515, "Y"=6178456.872776356}, {"X"=4531207.369890197, "Y"=6178456.738808704}, {"X"=4531204.963034085, "Y"=6178456.470882273}, {"X"=4531204.716938858, "Y"=6178456.208773792}, {"X"=4531204.506242221, "Y"=6178455.959187693}, {"X"=4531203.558565168, "Y"=6178455.905972362}, {"X"=4531202.700913063, "Y"=6178455.32054868}, {"X"=4531202.393884291, "Y"=6178455.338362789}, {"X"=4531202.0054720845, "Y"=6178455.405188011}, {"X"=4531201.509169189, "Y"=6178455.6088981405}, {"X"=4531200.994277919, "Y"=6178455.796307448}, {"X"=4531200.518341855, "Y"=6178456.036397454}, {"X"=4531198.533298231, "Y"=6178457.240298655}, {"X"=4531197.437331914, "Y"=6178458.029331279}, {"X"=4531196.355592065, "Y"=6178458.97899676}, {"X"=4531195.9071363555, "Y"=6178459.3357825605}, {"X"=4531195.300359756, "Y"=6178459.840787957}, {"X"=4531195.305777904, "Y"=6178460.095556019}, {"X"=4531194.58691523, "Y"=6178461.270838985}, {"X"=4531196.1067739725, "Y"=6178460.622036846}, {"X"=4531196.166984801, "Y"=6178460.721137047}, {"X"=4531196.136921037, "Y"=6178460.768852235}, {"X"=4531196.021917444, "Y"=6178460.825419938}, {"X"=4531195.8078312725, "Y"=6178460.924737332}, {"X"=4531195.385882864, "Y"=6178461.193649175}, {"X"=4531195.137287339, "Y"=6178461.290483773}, {"X"=4531194.630399219, "Y"=6178461.568248004}, {"X"=4531194.388027636, "Y"=6178461.735359617}, {"X"=4531194.101699417, "Y"=6178462.567674694}, {"X"=4531193.992113912, "Y"=6178462.8790101325}, {"X"=4531193.76574663, "Y"=6178463.226833953}, {"X"=4531193.664969111, "Y"=6178463.444034718}, {"X"=4531193.467776462, "Y"=6178463.734103757}, {"X"=4531193.253773695, "Y"=6178464.02795114}, {"X"=4531192.509932385, "Y"=6178464.72759357}, {"X"=4531192.326882534, "Y"=6178464.983765263}, {"X"=4531192.136080167, "Y"=6178465.733171325}, {"X"=4531192.073451645, "Y"=6178466.187543024}, {"X"=4531192.020520247, "Y"=6178466.557819762}, {"X"=4531192.076534677, "Y"=6178467.190312373}, {"X"=4531192.01915761, "Y"=6178467.51039121}, {"X"=4531191.834495636, "Y"=6178468.135543612}, {"X"=4531191.90804295, "Y"=6178468.38523712}, {"X"=4531191.855917442, "Y"=6178468.57102317}, {"X"=4531191.803791933, "Y"=6178468.756809216}, {"X"=4531191.563364835, "Y"=6178469.333059115}, {"X"=4531191.291901832, "Y"=6178469.75245429}, {"X"=4531190.724969863, "Y"=6178470.320176326}, {"X"=4531190.456091232, "Y"=6178470.575160005}, {"X"=4531190.169513414, "Y"=6178470.823882443}, {"X"=4531189.868792848, "Y"=6178471.106501837}, {"X"=4531189.042679781, "Y"=6178471.845111961}, {"X"=4531188.740181094, "Y"=6178472.107652034}, {"X"=4531188.389919483, "Y"=6178472.411645725}, {"X"=4531188.090088175, "Y"=6178472.704304305}, {"X"=4531187.428602893, "Y"=6178473.559501498}, {"X"=4531187.239661121, "Y"=6178474.523513481}, {"X"=4531185.889768906, "Y"=6178475.349131384}, {"X"=4531185.180272278, "Y"=6178475.662192495}, {"X"=4531183.691371847, "Y"=6178476.273309049}, {"X"=4531183.4544186, "Y"=6178476.69518506}, {"X"=4531183.604903009, "Y"=6178476.845669912}, {"X"=4531184.111789394, "Y"=6178476.5679095695}, {"X"=4531186.329106401, "Y"=6178476.438150704}, {"X"=4531186.769807618, "Y"=6178476.574601925}, {"X"=4531191.36576348, "Y"=6178476.975104507}, {"X"=4531192.0063251965, "Y"=6178476.851607449}, {"X"=4531191.868370715, "Y"=6178477.0362056075}, {"X"=4531191.632222962, "Y"=6178477.273592302}, {"X"=4531191.417330766, "Y"=6178477.557398377}, {"X"=4531191.457174578, "Y"=6178477.62011859}, {"X"=4531191.443031753, "Y"=6178477.654015556}, {"X"=4531191.527971299, "Y"=6178477.645163527}, {"X"=4531191.067068773, "Y"=6178477.86139137}, {"X"=4531190.096694444, "Y"=6178478.51979054}, {"X"=4531189.969326494, "Y"=6178478.630333359}, {"X"=4531189.836624006, "Y"=6178478.680638917}, {"X"=4531189.853434088, "Y"=6178478.676860611}, {"X"=4531189.902975247, "Y"=6178478.6554861395}, {"X"=4531190.216225832, "Y"=6178478.707951097}, {"X"=4531190.492382494, "Y"=6178478.922344166}, {"X"=4531190.753507225, "Y"=6178479.160594666}, {"X"=4531190.8933224315, "Y"=6178479.190605488}, {"X"=4531191.00574107, "Y"=6178479.298449748}, {"X"=4531191.173924478, "Y"=6178479.455196376}, {"X"=4531191.089956583, "Y"=6178479.668617567}, {"X"=4531192.149881182, "Y"=6178479.440624}, {"X"=4531192.553323351, "Y"=6178479.349944692}, {"X"=4531193.621085086, "Y"=6178478.8232473}, {"X"=4531194.08295944, "Y"=6178478.811588988}, {"X"=4531194.581121281, "Y"=6178478.822492746}, {"X"=4531194.722714726, "Y"=6178478.872582749}, {"X"=4531194.726271052, "Y"=6178478.912740986}, {"X"=4531194.751082888, "Y"=6178478.999318712}, {"X"=4531194.686509736, "Y"=6178479.044550614}, {"X"=4531194.569728123, "Y"=6178479.081038319}, {"X"=4531194.402433763, "Y"=6178478.934331035}, {"X"=4531193.964317197, "Y"=6178478.633467706}, {"X"=4531193.742147099, "Y"=6178478.447897628}, {"X"=4531193.359071229, "Y"=6178478.574956974}, {"X"=4531192.841514641, "Y"=6178478.732242771}, {"X"=4531192.435405168, "Y"=6178478.792803512}, {"X"=4531192.266415163, "Y"=6178478.820547042}, {"X"=4531191.145473723, "Y"=6178479.133930901}, {"X"=4531191.035804896, "Y"=6178479.250734952}, {"X"=4531190.910132516, "Y"=6178479.186827185}, {"X"=4531190.793351004, "Y"=6178479.223314872}, {"X"=4531190.6650939295, "Y"=6178479.323818126}, {"X"=4531190.536836865, "Y"=6178479.424321368}, {"X"=4531190.373181457, "Y"=6178479.512302125}, {"X"=4531190.15909582, "Y"=6178479.611617778}, {"X"=4531190.122808394, "Y"=6178479.589055759}, {"X"=4531189.955596661, "Y"=6178479.63687833}, {"X"=4531189.843260612, "Y"=6178479.723563695}, {"X"=4531189.764544732, "Y"=6178479.802692451}, {"X"=4531189.734480919, "Y"=6178479.850407218}, {"X"=4531189.630953175, "Y"=6178479.842958405}, {"X"=4531189.544235512, "Y"=6178479.831731294}, {"X"=4531189.44515321, "Y"=6178479.874480181}, {"X"=4531189.337180038, "Y"=6178479.816833674}, {"X"=4531189.108062546, "Y"=6178479.940006667}, {"X"=4531189.06296684, "Y"=6178480.011578797}, {"X"=4531188.960410779, "Y"=6178480.208699036}, {"X"=4531188.947963557, "Y"=6178480.0681455145}, {"X"=4531188.649910203, "Y"=6178480.380882081}, {"X"=4531188.535796023, "Y"=6178480.447488309}, {"X"=4531188.411095385, "Y"=6178480.588149576}, {"X"=4531188.346522347, "Y"=6178480.633381366}, {"X"=4531188.174058758, "Y"=6178480.815496103}, {"X"=4531188.141327695, "Y"=6178480.833092226}, {"X"=4531187.975894227, "Y"=6178480.900993779}, {"X"=4531187.941384996, "Y"=6178480.898510834}, {"X"=4531187.959973247, "Y"=6178480.914811604}, {"X"=4531187.910432113, "Y"=6178480.936186026}, {"X"=4531187.845052575, "Y"=6178481.165907678}, {"X"=4531187.784035892, "Y"=6178481.251297574}, {"X"=4531187.673560652, "Y"=6178481.552591261}, {"X"=4531187.697483402, "Y"=6178481.629129218}, {"X"=4531187.704596083, "Y"=6178481.709445466}, {"X"=4531187.686896932, "Y"=6178481.703184227}, {"X"=4531187.684229678, "Y"=6178481.673065634}, {"X"=4531187.645275026, "Y"=6178481.6203850275}, {"X"=4531187.624908609, "Y"=6178481.584005189}, {"X"=4531187.6213522665, "Y"=6178481.543847065}, {"X"=4531187.533745578, "Y"=6178481.522580401}, {"X"=4531187.379787694, "Y"=6178481.526466431}, {"X"=4531187.379787694, "Y"=6178481.526466431}, {"X"=4531187.445249799, "Y"=6178481.491274201}, {"X"=4531187.527521975, "Y"=6178481.452303686}, {"X"=4531187.655778934, "Y"=6178481.351800636}, {"X"=4531187.669921742, "Y"=6178481.317903749}, {"X"=4531187.717684698, "Y"=6178481.276450274}, {"X"=4531187.742413974, "Y"=6178481.168498372}, {"X"=4531187.800763396, "Y"=6178481.052989877}, {"X"=4531187.830827191, "Y"=6178481.005275161}, {"X"=4531187.812238947, "Y"=6178480.988974387}, {"X"=4531187.79098344, "Y"=6178480.9425550215}, {"X"=4531187.7706170175, "Y"=6178480.906175184}, {"X"=4531187.765282492, "Y"=6178480.845937989}, {"X"=4531187.731662349, "Y"=6178480.853494583}, {"X"=4531187.71129593, "Y"=6178480.817114751}, {"X"=4531187.7934855195, "Y"=6178480.583614793}, {"X"=4531188.244442415, "Y"=6178479.867893772}, {"X"=4531188.2806472145, "Y"=6178479.695926292}, {"X"=4531188.266504404, "Y"=6178479.729823208}, {"X"=4531188.227632344, "Y"=6178479.871672071}, {"X"=4531188.245331504, "Y"=6178479.877933305}, {"X"=4531188.2161568, "Y"=6178479.935687583}, {"X"=4531188.189649363, "Y"=6178480.023560467}, {"X"=4531188.210904881, "Y"=6178480.069979837}, {"X"=4531188.201207517, "Y"=6178480.15407442}, {"X"=4531188.218906679, "Y"=6178480.160335652}]  # 20200920 burim-3
  (unwired) cluster{"X":dbl, "Y":dbl}[] [{"X"=4531189.024901247, "Y"=6178479.968937709}, {"X"=4531189.140793614, "Y"=6178479.922410529}, {"X"=4531189.369911104, "Y"=6178479.799237533}, {"X"=4531189.721144613, "Y"=6178479.699814109}, {"X"=4531189.853847085, "Y"=6178479.649508607}, {"X"=4531190.88370759, "Y"=6178479.469229817}, {"X"=4531194.528188635, "Y"=6178479.192768817}, {"X"=4531196.095166773, "Y"=6178479.076074553}, {"X"=4531196.879100548, "Y"=6178479.022747226}, {"X"=4531198.1823697155, "Y"=6178478.832213253}, {"X"=4531199.6742713945, "Y"=6178479.029336632}, {"X"=4531200.278628806, "Y"=6178479.0778082805}, {"X"=4531202.734042382, "Y"=6178479.119806239}, {"X"=4531203.634758914, "Y"=6178479.029991464}, {"X"=4531204.553174814, "Y"=6178478.946437978}, {"X"=4531205.421160467, "Y"=6178478.874219427}, {"X"=4531206.087424596, "Y"=6178478.847340586}, {"X"=4531206.843073887, "Y"=6178478.861807829}, {"X"=4531207.829619984, "Y"=6178478.773180793}, {"X"=4531208.694857004, "Y"=6178478.476312651}, {"X"=4531209.681157538, "Y"=6178477.804092788}, {"X"=4531209.973878647, "Y"=6178477.431116413}, {"X"=4531210.248900546, "Y"=6178477.051878661}, {"X"=4531210.595608406, "Y"=6178476.707725614}, {"X"=4531210.860043622, "Y"=6178476.4025433315}, {"X"=4531210.889861566, "Y"=6178475.771235004}, {"X"=4531210.915398248, "Y"=6178475.478790694}, {"X"=4531211.695450017, "Y"=6178474.60717989}, {"X"=4531211.997950934, "Y"=6178474.344638677}, {"X"=4531212.317262051, "Y"=6178474.078319069}, {"X"=4531212.860918354, "Y"=6178472.860501966}, {"X"=4531213.394152205, "Y"=6178472.1058027055}, {"X"=4531213.767368098, "Y"=6178471.673774758}, {"X"=4531214.128219191, "Y"=6178471.295723215}, {"X"=4531214.643029188, "Y"=6178470.913785264}, {"X"=4531215.193237774, "Y"=6178470.544369738}, {"X"=4531215.5009912355, "Y"=6178470.147534006}, {"X"=4531216.327029055, "Y"=6178469.214386662}, {"X"=4531217.575907016, "Y"=6178468.022366559}, {"X"=4531218.011111873, "Y"=6178467.70951769}, {"X"=4531218.731118977, "Y"=6178467.127864759}, {"X"=4531219.059239212, "Y"=6178466.7674083235}, {"X"=4531219.336928843, "Y"=6178466.41828695}, {"X"=4531220.470803541, "Y"=6178465.282831962}, {"X"=4531220.869721097, "Y"=6178464.947420141}, {"X"=4531221.3181802705, "Y"=6178464.590633356}, {"X"=4531222.214045182, "Y"=6178463.477955396}, {"X"=4531222.933970839, "Y"=6178462.701768192}, {"X"=4531223.295711876, "Y"=6178462.333753782}, {"X"=4531223.657452951, "Y"=6178461.965739275}, {"X"=4531224.538368582, "Y"=6178461.071449561}, {"X"=4531225.056571771, "Y"=6178460.340602083}, {"X"=4531225.826846314, "Y"=6178459.3585453}, {"X"=4531226.270778315, "Y"=6178458.757025854}, {"X"=4531228.089100469, "Y"=6178456.638318795}, {"X"=4531228.046424221, "Y"=6178456.1564130625}, {"X"=4531227.227891228, "Y"=6178456.012729765}, {"X"=4531226.749202252, "Y"=6178456.028169088}, {"X"=4531226.286434477, "Y"=6178456.029790269}, {"X"=4531225.791824421, "Y"=6178456.059047765}, {"X"=4531223.721331555, "Y"=6178456.10461287}, {"X"=4531223.187766663, "Y"=6178456.0811891975}, {"X"=4531222.69137868, "Y"=6178456.090367399}, {"X"=4531218.368067964, "Y"=6178456.058648482}, {"X"=4531215.709137241, "Y"=6178456.0419283705}, {"X"=4531215.187131444, "Y"=6178456.1490206625}, {"X"=4531214.6943005845, "Y"=6178456.198357753}, {"X"=4531212.951207607, "Y"=6178456.262490641}, {"X"=4531212.40091638, "Y"=6178456.437377693}, {"X"=4531210.435094997, "Y"=6178457.084027206}, {"X"=4531209.267995648, "Y"=6178457.069891132}, {"X"=4531208.8476578165, "Y"=6178456.969820701}, {"X"=4531207.351384872, "Y"=6178456.917039323}, {"X"=4531205.285344398, "Y"=6178457.01280454}, {"X"=4531204.727941156, "Y"=6178457.107374322}, {"X"=4531204.182985723, "Y"=6178457.342498767}, {"X"=4531203.79465667, "Y"=6178457.603854876}, {"X"=4531203.390406607, "Y"=6178457.879028972}, {"X"=4531202.987045717, "Y"=6178458.164242608}, {"X"=4531202.109526927, "Y"=6178458.709624942}, {"X"=4531201.655735695, "Y"=6178459.006173636}, {"X"=4531201.201944525, "Y"=6178459.302722244}, {"X"=4531200.765852696, "Y"=6178459.605531941}, {"X"=4531200.260742047, "Y"=6178459.9033760475}, {"X"=4531199.7565205945, "Y"=6178460.211259656}, {"X"=4531199.438989132, "Y"=6178460.497659723}, {"X"=4531199.072888672, "Y"=6178461.010004938}, {"X"=4531198.937601528, "Y"=6178461.224723443}, {"X"=4531198.500704026, "Y"=6178461.712023724}, {"X"=4531198.270779874, "Y"=6178462.019689773}, {"X"=4531197.061754517, "Y"=6178463.274427918}, {"X"=4531196.67876097, "Y"=6178463.5960201}, {"X"=4531195.94639426, "Y"=6178464.231647407}, {"X"=4531195.136200883, "Y"=6178464.956443402}, {"X"=4531194.600138173, "Y"=6178465.291961507}, {"X"=4531194.149015275, "Y"=6178465.618627125}, {"X"=4531192.972805475, "Y"=6178467.050295575}, {"X"=4531191.496432121, "Y"=6178467.996501925}, {"X"=4531191.395820698, "Y"=6178468.6027622875}, {"X"=4531191.754416784, "Y"=6178469.167243971}, {"X"=4531191.829742241, "Y"=6178469.437016584}, {"X"=4531191.687425391, "Y"=6178469.765947495}, {"X"=4531191.403514802, "Y"=6178470.044788794}, {"X"=4531190.006747082, "Y"=6178470.92190334}, {"X"=4531188.593086821, "Y"=6178471.608265689}, {"X"=4531188.247270787, "Y"=6178471.962457186}, {"X"=4531188.120875055, "Y"=6178472.277569592}, {"X"=4531188.053160451, "Y"=6178473.255291844}, {"X"=4531188.01259331, "Y"=6178473.571591496}, {"X"=4531187.988836232, "Y"=6178473.884112789}, {"X"=4531187.948269044, "Y"=6178474.200412402}, {"X"=4531187.910369151, "Y"=6178474.546830607}, {"X"=4531187.044269077, "Y"=6178476.963444959}, {"X"=4531186.647133752, "Y"=6178477.3189308075}, {"X"=4531186.724567966, "Y"=6178478.386899571}, {"X"=4531187.121786068, "Y"=6178478.225943374}, {"X"=4531188.072930392, "Y"=6178478.124792789}, {"X"=4531189.053001488, "Y"=6178477.382299101}, {"X"=4531190.219121024, "Y"=6178477.191871992}, {"X"=4531190.8474006085, "Y"=6178477.316880768}, {"X"=4531191.173098596, "Y"=6178477.509899318}, {"X"=4531191.252868845, "Y"=6178477.829869464}, {"X"=4531190.567376832, "Y"=6178478.413997857}, {"X"=4531190.0153112905, "Y"=6178478.5688007185}, {"X"=4531189.538405336, "Y"=6178478.60431659}, {"X"=4531189.407398402, "Y"=6178478.480171638}, {"X"=4531189.502924346, "Y"=6178478.397264526}, {"X"=4531189.517067156, "Y"=6178478.363367595}, {"X"=4531189.697449958, "Y"=6178478.07707884}, {"X"=4531189.728402851, "Y"=6178478.039403586}, {"X"=4531191.843082795, "Y"=6178477.912237325}, {"X"=4531191.779398787, "Y"=6178477.967508781}, {"X"=4531191.716603865, "Y"=6178478.032819781}, {"X"=4531191.7033501305, "Y"=6178478.076756295}, {"X"=4531191.754669494, "Y"=6178478.075460904}, {"X"=4531191.789178761, "Y"=6178478.07794383}, {"X"=4531191.826355298, "Y"=6178478.110545404}, {"X"=4531191.997123472, "Y"=6178478.102880929}, {"X"=4531192.0289654825, "Y"=6178478.075245205}, {"X"=4531192.408484912, "Y"=6178477.908027585}, {"X"=4531192.607538775, "Y"=6178477.832569163}, {"X"=4531192.9180397, "Y"=6178477.660385651}, {"X"=4531193.01801119, "Y"=6178477.627676205}, {"X"=4531193.101172581, "Y"=6178477.598745075}, {"X"=4531193.201144077, "Y"=6178477.566035621}, {"X"=4531193.486026644, "Y"=6178477.491764693}, {"X"=4531193.540013286, "Y"=6178477.520587969}, {"X"=4531193.629398301, "Y"=6178477.561933729}, {"X"=4531193.785134622, "Y"=6178477.578126672}, {"X"=4531194.060319813, "Y"=6178477.587950529}, {"X"=4531194.19924604, "Y"=6178477.607921798}, {"X"=4531194.284185625, "Y"=6178477.599069774}, {"X"=4531194.353204202, "Y"=6178477.604035629}, {"X"=4531194.423111863, "Y"=6178477.619041043}, {"X"=4531194.459399322, "Y"=6178477.641603093}, {"X"=4531194.462955662, "Y"=6178477.681761331}, {"X"=4531194.466512003, "Y"=6178477.72191957}, {"X"=4531194.518720474, "Y"=6178477.730663746}, {"X"=4531194.625804672, "Y"=6178477.7782707745}, {"X"=4531194.734667042, "Y"=6178477.845956929}, {"X"=4531194.688682166, "Y"=6178477.90748967}, {"X"=4531194.789542768, "Y"=6178477.884819791}, {"X"=4531194.937359841, "Y"=6178478.005186694}, {"X"=4531195.011712914, "Y"=6178478.0703899255}, {"X"=4531195.047111284, "Y"=6178478.082912429}, {"X"=4531195.063032303, "Y"=6178478.06909455}, {"X"=4531195.063921385, "Y"=6178478.079134112}, {"X"=4531195.16389292, "Y"=6178478.046424675}, {"X"=4531195.19751313, "Y"=6178478.038868048}, {"X"=4531195.247943432, "Y"=6178478.027533113}, {"X"=4531195.334661199, "Y"=6178478.038760231}, {"X"=4531195.367392322, "Y"=6178478.021164046}]  # 20200920 burim-2
  (unwired) cluster{"X":dbl, "Y":dbl}[] [{"X"=4531192.172254518, "Y"=6178477.950884427}, {"X"=4531192.285479729, "Y"=6178477.874238477}, {"X"=4531192.411958685, "Y"=6178477.7536559915}, {"X"=4531193.3948634565, "Y"=6178477.430339825}, {"X"=4531194.8238045275, "Y"=6178477.303712808}, {"X"=4531195.60596018, "Y"=6178477.23030582}, {"X"=4531197.831283162, "Y"=6178477.190905031}, {"X"=4531198.479847411, "Y"=6178477.157764238}, {"X"=4531200.803282672, "Y"=6178476.871044792}, {"X"=4531202.676484059, "Y"=6178476.921028848}, {"X"=4531205.416618444, "Y"=6178476.499693098}, {"X"=4531206.099692973, "Y"=6178476.469035389}, {"X"=4531207.421635327, "Y"=6178476.48933225}, {"X"=4531207.879065608, "Y"=6178476.42747596}, {"X"=4531208.36300371, "Y"=6178476.277746148}, {"X"=4531208.847830933, "Y"=6178476.138055908}, {"X"=4531209.548523046, "Y"=6178475.919128562}, {"X"=4531210.833125568, "Y"=6178475.51776158}, {"X"=4531211.616090724, "Y"=6178475.259863131}, {"X"=4531213.312946614, "Y"=6178474.6736807525}, {"X"=4531213.768517382, "Y"=6178474.397213681}, {"X"=4531214.732592756, "Y"=6178473.47400039}, {"X"=4531215.080190111, "Y"=6178473.139885966}, {"X"=4531215.460518798, "Y"=6178472.788175125}, {"X"=4531215.943486765, "Y"=6178472.433873379}, {"X"=4531216.919202614, "Y"=6178471.835705624}, {"X"=4531217.325232342, "Y"=6178471.58061249}, {"X"=4531217.903563232, "Y"=6178470.754338925}, {"X"=4531218.3466056045, "Y"=6178470.142783957}, {"X"=4531218.646439895, "Y"=6178469.850122707}, {"X"=4531218.82771374, "Y"=6178469.573870302}, {"X"=4531218.991288323, "Y"=6178469.291356563}, {"X"=4531219.220325571, "Y"=6178468.9736499945}, {"X"=4531219.8827897925, "Y"=6178468.323015164}, {"X"=4531220.077317608, "Y"=6178468.002825483}, {"X"=4531220.036502491, "Y"=6178467.735533033}, {"X"=4531220.075853423, "Y"=6178466.631062238}, {"X"=4531220.235871674, "Y"=6178466.308389446}, {"X"=4531220.464908921, "Y"=6178465.99068239}, {"X"=4531221.273248552, "Y"=6178465.051270751}, {"X"=4531222.056776412, "Y"=6178464.025279861}, {"X"=4531222.396372686, "Y"=6178463.600806138}, {"X"=4531223.503411304, "Y"=6178461.77509362}, {"X"=4531223.577600251, "Y"=6178461.451232713}, {"X"=4531223.654456428, "Y"=6178461.15749082}, {"X"=4531223.695913951, "Y"=6178460.851226377}, {"X"=4531223.588746596, "Y"=6178460.609086748}, {"X"=4531223.038289529, "Y"=6178460.394908377}, {"X"=4531222.725036301, "Y"=6178460.34244384}, {"X"=4531222.043653754, "Y"=6178460.198651705}, {"X"=4531221.79319603, "Y"=6178460.080875152}, {"X"=4531221.509117848, "Y"=6178459.970655465}, {"X"=4531221.209118525, "Y"=6178459.874253907}, {"X"=4531220.873720572, "Y"=6178459.765329881}, {"X"=4531220.519734208, "Y"=6178459.64010497}, {"X"=4531219.807316021, "Y"=6178459.3394569075}, {"X"=4531218.050720693, "Y"=6178458.86392827}, {"X"=4531216.519853841, "Y"=6178458.614129987}, {"X"=4531215.674732223, "Y"=6178458.363789538}, {"X"=4531214.75622884, "Y"=6178458.252817324}, {"X"=4531214.170456079, "Y"=6178458.220649713}, {"X"=4531213.016610021, "Y"=6178458.1625758195}, {"X"=4531212.531698616, "Y"=6178458.107737698}, {"X"=4531212.014945064, "Y"=6178458.080535778}, {"X"=4531210.957514985, "Y"=6178457.949593326}, {"X"=4531210.309836433, "Y"=6178457.992777574}, {"X"=4531208.326233964, "Y"=6178458.438633115}, {"X"=4531207.650270089, "Y"=6178458.549611997}, {"X"=4531206.997340306, "Y"=6178458.727089811}, {"X"=4531206.299314793, "Y"=6178458.976140626}, {"X"=4531205.586257464, "Y"=6178459.249049017}, {"X"=4531204.922741668, "Y"=6178459.500582404}, {"X"=4531204.240637578, "Y"=6178459.735814891}, {"X"=4531203.575343774, "Y"=6178459.967268877}, {"X"=4531201.33183938, "Y"=6178460.963035614}, {"X"=4531200.452542792, "Y"=6178461.488337481}, {"X"=4531199.9288438205, "Y"=6178461.769880375}, {"X"=4531199.383000062, "Y"=6178461.994964011}, {"X"=4531198.210818546, "Y"=6178462.5041815}, {"X"=4531197.514572887, "Y"=6178462.773310179}, {"X"=4531196.534582699, "Y"=6178463.710342408}, {"X"=4531195.931445486, "Y"=6178464.450035426}, {"X"=4531195.442256568, "Y"=6178464.734060204}, {"X"=4531195.021197344, "Y"=6178465.0130109005}, {"X"=4531194.156045099, "Y"=6178465.504413416}, {"X"=4531193.253716351, "Y"=6178465.9632141655}, {"X"=4531193.018457816, "Y"=6178466.210641808}, {"X"=4531192.790312228, "Y"=6178466.538385953}, {"X"=4531192.122685636, "Y"=6178467.517839632}, {"X"=4531191.859141629, "Y"=6178467.83306115}, {"X"=4531191.559310067, "Y"=6178468.125720667}, {"X"=4531191.228525659, "Y"=6178468.456055547}, {"X"=4531190.915440501, "Y"=6178468.79265153}, {"X"=4531190.421083745, "Y"=6178469.4054976525}, {"X"=4531190.017001325, "Y"=6178470.069728596}, {"X"=4531189.741175928, "Y"=6178470.633455561}, {"X"=4531189.702470089, "Y"=6178471.164364505}, {"X"=4531189.59021706, "Y"=6178471.445580124}, {"X"=4531188.999136827, "Y"=6178473.482961793}, {"X"=4531188.061577024, "Y"=6178474.318295965}, {"X"=4531187.701618197, "Y"=6178474.706383894}, {"X"=4531187.460219085, "Y"=6178475.078062939}, {"X"=4531187.1127906125, "Y"=6178475.8012337135}, {"X"=4531188.494215864, "Y"=6178476.299647906}, {"X"=4531189.872808392, "Y"=6178476.378884667}, {"X"=4531190.164886286, "Y"=6178476.579459694}, {"X"=4531190.1218168745, "Y"=6178477.254700084}, {"X"=4531190.147517886, "Y"=6178477.351317219}, {"X"=4531190.075832075, "Y"=6178477.316232765}, {"X"=4531189.628824399, "Y"=6178476.914974731}, {"X"=4531189.4694490405, "Y"=6178476.664094075}, {"X"=4531190.193337309, "Y"=6178476.900725166}, {"X"=4531190.812726004, "Y"=6178476.925338404}, {"X"=4531191.438255739, "Y"=6178476.825698755}, {"X"=4531192.021274462, "Y"=6178476.633220208}, {"X"=4531192.473368856, "Y"=6178476.511126412}, {"X"=4531192.84674736, "Y"=6178476.468161532}, {"X"=4531194.301306903, "Y"=6178476.243621304}, {"X"=4531194.302195992, "Y"=6178476.253660865}, {"X"=4531194.407502057, "Y"=6178476.281188726}, {"X"=4531194.529618229, "Y"=6178476.304938269}, {"X"=4531194.565905702, "Y"=6178476.327500306}, {"X"=4531194.760596821, "Y"=6178476.396373929}, {"X"=4531194.867681063, "Y"=6178476.4439809285}, {"X"=4531194.90574671, "Y"=6178476.486622101}, {"X"=4531194.943812361, "Y"=6178476.5292632645}, {"X"=4531194.982767095, "Y"=6178476.581943995}, {"X"=4531195.004911723, "Y"=6178476.63840305}, {"X"=4531195.082821187, "Y"=6178476.743764519}, {"X"=4531195.119997737, "Y"=6178476.776366131}, {"X"=4531195.158952467, "Y"=6178476.829046864}, {"X"=4531195.180208006, "Y"=6178476.875466362}, {"X"=4531195.183764351, "Y"=6178476.915624613}, {"X"=4531195.220134336, "Y"=6178477.132716679}, {"X"=4531195.207769663, "Y"=6178477.186692812}, {"X"=4531195.149420099, "Y"=6178477.302201706}, {"X"=4531195.120245312, "Y"=6178477.3599561555}, {"X"=4531195.025608287, "Y"=6178477.452902989}, {"X"=4531194.977845227, "Y"=6178477.49435662}, {"X"=4531194.9159393255, "Y"=6178477.569707253}, {"X"=4531194.837223323, "Y"=6178477.6488362}, {"X"=4531194.757618234, "Y"=6178477.71792558}, {"X"=4531194.725776199, "Y"=6178477.745561326}, {"X"=4531194.758507318, "Y"=6178477.727965142}, {"X"=4531194.588628131, "Y"=6178477.745669164}, {"X"=4531194.115278068, "Y"=6178477.821343292}, {"X"=4531193.183362322, "Y"=6178477.365244511}, {"X"=4531193.361078111, "Y"=6178477.048836683}, {"X"=4531193.276221112, "Y"=6178477.252218609}, {"X"=4531193.542763095, "Y"=6178477.745236524}, {"X"=4531193.426064045, "Y"=6178477.976254157}, {"X"=4531192.416816901, "Y"=6178478.776502722}, {"X"=4531192.593973703, "Y"=6178479.228174716}, {"X"=4531192.84782075, "Y"=6178478.997049441}, {"X"=4531193.045013939, "Y"=6178478.70698217}, {"X"=4531193.411114648, "Y"=6178478.194641449}, {"X"=4531193.185553247, "Y"=6178478.357972908}, {"X"=4531192.763522719, "Y"=6178478.432351564}, {"X"=4531191.844860973, "Y"=6178477.932316427}, {"X"=4531191.359063921, "Y"=6178477.867436871}, {"X"=4531190.919334335, "Y"=6178477.9355543805}, {"X"=4531190.426672517, "Y"=6178478.373947526}, {"X"=4531190.20466767, "Y"=6178478.57743703}, {"X"=4531189.86863122, "Y"=6178479.0420624325}, {"X"=4531189.891664924, "Y"=6178479.108560925}, {"X"=4531189.846569206, "Y"=6178479.180133095}, {"X"=4531189.81472722, "Y"=6178479.207768787}, {"X"=4531189.764296975, "Y"=6178479.219103704}]  # 20200920 burim-1
  (unwired) cluster{"X":dbl, "Y":dbl}[] [{"X"=4947391.932492469, "Y"=5830656.686136119}, {"X"=4947391.930480022, "Y"=5830656.662126245}, {"X"=4947391.985527909, "Y"=5830656.620670592}, {"X"=4947392.022561919, "Y"=5830656.597035126}, {"X"=4947392.039569586, "Y"=5830656.567209994}, {"X"=4947392.056577247, "Y"=5830656.537384859}, {"X"=4947392.094617479, "Y"=5830656.525754328}, {"X"=4947392.093611255, "Y"=5830656.513749392}, {"X"=4947392.031519798, "Y"=5830656.471170505}, {"X"=4947391.854301434, "Y"=5830656.451478253}, {"X"=4947391.52190349, "Y"=5830656.442293321}, {"X"=4947391.112418891, "Y"=5830656.444364526}, {"X"=4947390.665900317, "Y"=5830656.470071211}, {"X"=4947390.179329113, "Y"=5830656.483398585}, {"X"=4947389.652705268, "Y"=5830656.484346658}, {"X"=4947389.146107786, "Y"=5830656.491484427}, {"X"=4947388.557392553, "Y"=5830656.44985374}, {"X"=4947387.952675952, "Y"=5830656.450053142}, {"X"=4947387.405019688, "Y"=5830656.432806794}, {"X"=4947386.779270603, "Y"=5830656.41481172}, {"X"=4947386.250634508, "Y"=5830656.391750194}, {"X"=4947385.759032388, "Y"=5830656.345053262}, {"X"=4947385.210370018, "Y"=5830656.315802176}, {"X"=4947384.660701445, "Y"=5830656.274546223}, {"X"=4947384.0920128105, "Y"=5830656.239105598}, {"X"=4947383.574347018, "Y"=5830656.1141897645}, {"X"=4947383.092708918, "Y"=5830655.953633639}, {"X"=4947382.683126165, "Y"=5830655.721796868}, {"X"=4947382.3085648175, "Y"=5830655.442314905}, {"X"=4947382.085157846, "Y"=5830655.104305866}, {"X"=4947381.860744583, "Y"=5830654.754291957}, {"X"=4947381.823513361, "Y"=5830654.310110526}, {"X"=4947381.863368684, "Y"=5830653.854672829}, {"X"=4947382.036364585, "Y"=5830653.358528052}, {"X"=4947382.364539945, "Y"=5830652.8518755715}, {"X"=4947382.86590866, "Y"=5830652.316895133}, {"X"=4947383.445370343, "Y"=5830651.782663145}, {"X"=4947384.163004083, "Y"=5830651.267748461}, {"X"=4947384.9056955855, "Y"=5830650.819047802}, {"X"=4947385.692464968, "Y"=5830650.430745928}, {"X"=4947386.463233151, "Y"=5830650.084274017}, {"X"=4947387.258052849, "Y"=5830649.79201135}, {"X"=4947388.09393167, "Y"=5830649.524132801}, {"X"=4947388.877781532, "Y"=5830649.333724819}, {"X"=4947389.666662741, "Y"=5830649.203341524}, {"X"=4947390.499621791, "Y"=5830649.133357282}, {"X"=4947391.396685033, "Y"=5830649.129961779}, {"X"=4947392.334807365, "Y"=5830649.150950607}, {"X"=4947393.229858339, "Y"=5830649.123545413}, {"X"=4947393.911662947, "Y"=5830649.112088875}, {"X"=4947394.342180851, "Y"=5830649.1282115625}, {"X"=4947394.538419669, "Y"=5830649.142088225}, {"X"=4947394.795743851, "Y"=5830649.186538804}, {"X"=4947395.169201372, "Y"=5830649.220107476}, {"X"=4947395.718871361, "Y"=5830649.261363214}, {"X"=4947396.367667035, "Y"=5830649.321562338}, {"X"=4947397.017468983, "Y"=5830649.393766495}, {"X"=4947397.64623836, "Y"=5830649.447776102}, {"X"=4947398.333074458, "Y"=5830649.496344841}, {"X"=4947399.119036281, "Y"=5830649.563857035}, {"X"=4947399.979066353, "Y"=5830649.584098177}, {"X"=4947400.801056182, "Y"=5830649.615970033}, {"X"=4947401.58399954, "Y"=5830649.6474676}, {"X"=4947402.444029851, "Y"=5830649.667709047}, {"X"=4947403.420193702, "Y"=5830649.677068783}, {"X"=4947404.397363891, "Y"=5830649.698433641}, {"X"=4947405.429582299, "Y"=5830649.678342745}, {"X"=4947406.521880015, "Y"=5830649.676821082}, {"X"=4947407.577143727, "Y"=5830649.698935162}, {"X"=4947408.592354782, "Y"=5830649.708669969}, {"X"=4947409.530478998, "Y"=5830649.729661073}, {"X"=4947410.448576922, "Y"=5830649.744462576}, {"X"=4947411.462782132, "Y"=5830649.742192747}, {"X"=4947412.437940881, "Y"=5830649.739548622}, {"X"=4947413.4141059425, "Y"=5830649.748909623}, {"X"=4947414.299194853, "Y"=5830649.835367304}, {"X"=4947415.20229786, "Y"=5830649.904004808}, {"X"=4947415.994298233, "Y"=5830650.043549257}, {"X"=4947416.637155494, "Y"=5830650.265631228}, {"X"=4947417.131875755, "Y"=5830650.582255716}, {"X"=4947417.479465165, "Y"=5830651.005427719}, {"X"=4947417.696931547, "Y"=5830651.505321832}, {"X"=4947417.722183337, "Y"=5830652.039358625}, {"X"=4947417.577259339, "Y"=5830652.637737832}, {"X"=4947417.314189334, "Y"=5830653.22298841}, {"X"=4947416.8538740035, "Y"=5830653.782356263}, {"X"=4947416.351493613, "Y"=5830654.305334367}, {"X"=4947415.708928653, "Y"=5830654.784983941}, {"X"=4947414.986258307, "Y"=5830655.2398743015}, {"X"=4947414.126422039, "Y"=5830655.687451198}, {"X"=4947413.20147595, "Y"=5830656.056433598}, {"X"=4947412.211420065, "Y"=5830656.346821578}, {"X"=4947411.273394008, "Y"=5830656.559738737}, {"X"=4947410.460459894, "Y"=5830656.635909145}, {"X"=4947409.733571083, "Y"=5830656.574958365}, {"X"=4947408.94760942, "Y"=5830656.5074434355}, {"X"=4947408.140615267, "Y"=5830656.42173388}, {"X"=4947407.301617987, "Y"=5830656.41968489}, {"X"=4947406.554703039, "Y"=5830656.352544759}, {"X"=4947405.597560161, "Y"=5830656.337367544}, {"X"=4947404.605395677, "Y"=5830656.369835897}, {"X"=4947403.689311944, "Y"=5830656.379043335}, {"X"=4947402.714155471, "Y"=5830656.381686694}, {"X"=4947401.859157224, "Y"=5830656.421468457}, {"X"=4947401.218411704, "Y"=5830656.457307312}, {"X"=4947400.462539189, "Y"=5830656.516032777}, {"X"=4947399.762720969, "Y"=5830656.545307559}, {"X"=4947398.983803636, "Y"=5830656.561828536}, {"X"=4947398.281973146, "Y"=5830656.5670935}, {"X"=4947397.424963016, "Y"=5830656.582865737}, {"X"=4947396.624007158, "Y"=5830656.569187319}, {"X"=4947395.765991, "Y"=5830656.572954774}, {"X"=4947395.102201046, "Y"=5830656.566589496}, {"X"=4947394.749776637, "Y"=5830656.551214723}, {"X"=4947394.37933835, "Y"=5830656.553660172}, {"X"=4947394.203126152, "Y"=5830656.545972805}, {"X"=4947394.164079692, "Y"=5830656.545598378}, {"X"=4947394.164079692, "Y"=5830656.545598378}, {"X"=4947394.145059575, "Y"=5830656.5514136385}, {"X"=4947394.126039456, "Y"=5830656.557228906}, {"X"=4947394.1060131155, "Y"=5830656.551039222}, {"X"=4947394.086992989, "Y"=5830656.556854483}, {"X"=4947394.086992989, "Y"=5830656.556854483}, {"X"=4947393.715548504, "Y"=5830656.547295019}, {"X"=4947393.052764943, "Y"=5830656.552934864}, {"X"=4947392.154696496, "Y"=5830656.544323351}, {"X"=4947391.43183405, "Y"=5830656.53139431}, {"X"=4947391.024361923, "Y"=5830656.557475373}, {"X"=4947390.909235029, "Y"=5830656.580362022}, {"X"=4947390.871194815, "Y"=5830656.591992544}, {"X"=4947390.87220104, "Y"=5830656.603997477}, {"X"=4947390.854187151, "Y"=5830656.621817677}, {"X"=4947390.853180924, "Y"=5830656.609812743}, {"X"=4947390.853180924, "Y"=5830656.609812743}]  # pusan poly 0813
  (unwired) cluster{"X":dbl, "Y":dbl}[] [{"X"=4947397.140765152, "Y"=5830656.916008943}, {"X"=4947397.140765152, "Y"=5830656.916008943}, {"X"=4947397.121745022, "Y"=5830656.921824197}, {"X"=4947397.101718679, "Y"=5830656.9156345045}, {"X"=4947397.063678414, "Y"=5830656.92726502}, {"X"=4947397.043652072, "Y"=5830656.921075323}, {"X"=4947397.024631942, "Y"=5830656.92689058}, {"X"=4947397.024631942, "Y"=5830656.92689058}, {"X"=4947397.024631942, "Y"=5830656.92689058}, {"X"=4947397.023625729, "Y"=5830656.914885628}, {"X"=4947397.199837968, "Y"=5830656.922573082}, {"X"=4947397.43512303, "Y"=5830656.936824687}, {"X"=4947397.475175711, "Y"=5830656.949204081}, {"X"=4947397.455149368, "Y"=5830656.943014387}, {"X"=4947396.63316101, "Y"=5830656.911141239}, {"X"=4947395.031249629, "Y"=5830656.883784516}, {"X"=4947393.5094439145, "Y"=5830656.881186858}, {"X"=4947392.376090536, "Y"=5830656.858323781}, {"X"=4947391.55510889, "Y"=5830656.838456156}, {"X"=4947390.7561661005, "Y"=5830656.848788159}, {"X"=4947390.034310053, "Y"=5830656.847864113}, {"X"=4947389.272401408, "Y"=5830656.8345608115}, {"X"=4947388.392347302, "Y"=5830656.808129477}, {"X"=4947387.669485233, "Y"=5830656.795200737}, {"X"=4947386.887550475, "Y"=5830656.775708027}, {"X"=4947386.044530563, "Y"=5830656.725641541}, {"X"=4947385.07833405, "Y"=5830656.602422564}, {"X"=4947384.182180527, "Y"=5830656.38391324}, {"X"=4947383.587329651, "Y"=5830656.036345051}, {"X"=4947383.196668446, "Y"=5830655.564784444}, {"X"=4947382.970144199, "Y"=5830654.956852066}, {"X"=4947383.005876078, "Y"=5830654.219486117}, {"X"=4947383.325902977, "Y"=5830653.3828858165}, {"X"=4947383.739017822, "Y"=5830652.493198976}, {"X"=4947384.479598042, "Y"=5830651.786580115}, {"X"=4947385.481527273, "Y"=5830651.172430929}, {"X"=4947386.550579606, "Y"=5830650.660884811}, {"X"=4947387.705775168, "Y"=5830650.246126577}, {"X"=4947388.835005754, "Y"=5830649.987058049}, {"X"=4947390.031359405, "Y"=5830649.830592981}, {"X"=4947391.332876351, "Y"=5830649.765100905}, {"X"=4947392.716511511, "Y"=5830649.748377457}, {"X"=4947394.041074038, "Y"=5830649.725090241}, {"X"=4947395.210456962, "Y"=5830649.712310792}, {"X"=4947396.420899045, "Y"=5830649.723915781}, {"X"=4947397.634359998, "Y"=5830649.771535861}, {"X"=4947398.728669068, "Y"=5830649.794023103}, {"X"=4947399.859006149, "Y"=5830649.780869964}, {"X"=4947401.108495469, "Y"=5830649.792850075}, {"X"=4947402.397031535, "Y"=5830649.805204782}, {"X"=4947403.763660925, "Y"=5830649.81830849}, {"X"=4947405.225391419, "Y"=5830649.802335968}, {"X"=4947406.650088039, "Y"=5830649.809999293}, {"X"=4947408.01369953, "Y"=5830649.787088738}, {"X"=4947409.280197907, "Y"=5830649.769244852}, {"X"=4947410.606775687, "Y"=5830649.769970313}, {"X"=4947411.896319492, "Y"=5830649.79433159}, {"X"=4947413.088750085, "Y"=5830649.823759506}, {"X"=4947414.319221254, "Y"=5830649.841557039}, {"X"=4947415.494644366, "Y"=5830649.900810694}, {"X"=4947416.537932304, "Y"=5830650.012776601}, {"X"=4947417.281927788, "Y"=5830650.277812436}, {"X"=4947417.8037177455, "Y"=5830650.684662035}, {"X"=4947418.143354913, "Y"=5830651.245704836}, {"X"=4947418.147671333, "Y"=5830651.995457877}, {"X"=4947417.851688948, "Y"=5830652.886275241}, {"X"=4947417.186273139, "Y"=5830653.791542069}, {"X"=4947416.296542553, "Y"=5830654.580700927}, {"X"=4947415.314632557, "Y"=5830655.201040073}, {"X"=4947414.133465299, "Y"=5830655.771486305}, {"X"=4947412.792087455, "Y"=5830656.292414191}, {"X"=4947411.374532018, "Y"=5830656.602692522}, {"X"=4947409.979924542, "Y"=5830656.721265353}, {"X"=4947408.593269475, "Y"=5830656.701968151}, {"X"=4947407.221610036, "Y"=5830656.628835995}, {"X"=4947405.811910477, "Y"=5830656.567334638}, {"X"=4947404.421231292, "Y"=5830656.50001832}, {"X"=4947403.073623623, "Y"=5830656.481096663}, {"X"=4947401.8241355335, "Y"=5830656.4691138845}, {"X"=4947400.555627499, "Y"=5830656.462946556}, {"X"=4947399.268099511, "Y"=5830656.462594706}, {"X"=4947398.114718899, "Y"=5830656.433541202}, {"X"=4947397.194611097, "Y"=5830656.394729533}, {"X"=4947396.609920161, "Y"=5830656.401117986}, {"X"=4947396.433707921, "Y"=5830656.393430567}, {"X"=4947396.415694006, "Y"=5830656.41125078}, {"X"=4947396.434714136, "Y"=5830656.405435518}, {"X"=4947396.453734259, "Y"=5830656.399620261}, {"X"=4947396.491774522, "Y"=5830656.387989743}, {"X"=4947396.5118008675, "Y"=5830656.394179432}, {"X"=4947396.531827211, "Y"=5830656.400369123}, {"X"=4947396.550847346, "Y"=5830656.39455386}, {"X"=4947396.570873691, "Y"=5830656.400743557}]  # pusan poly 0812
  n1 = flat-sequence {
    tunnel: [w10] -> w1
    frame #0 {
      n2 = call "fgv_gps_config.vi"("cmd"=enum16{"read", "write"}."write", "GNSS cfg"="GNSS cfg") -> ("error out"=w10:errorcluster)  [unwired: 8 in, 1 out]
    }
  }
  n3 = call "fgv_232_F9P.vi"("cmd"=enum16{"init", "read", "write", "close"}."init", "error in"=w1) -> ("error out"=w5:errorcluster)  [unwired: 7 in, 2 out]
  n4 = while {
    shift-right: [w29] -> _
    shift-left: "" -> [w30]
    shift-right: [w24] -> _
    shift-left: cluster{dbl, dbl}[] [] -> [w12]
    tunnel: w5 -> [w26]
    tunnel: [w20] -> w3
    i -> [w21]
    stop <- w18 stop-if-true
    n5 = call "fgv_232_F9P.vi"("cmd"=enum16{"init", "read", "write", "close"}."read", "error in"=w26) -> ("error out"=w20:errorcluster, "byte n"=→"buff-n":u32, "read_buffer"=w15:string)  [unwired: 7 in]
    "error out" <- w20
    n6 = Not Equal?(x=w15, y="") -> (x != y?=→"data check":bool)
    n7 = call "sub_ubx-packet-final.vi"("read_buffer"=w15) -> ("ubx pk arr"=→"ubx arr":T1[])  [unwired: 10 in]
    n8 = call "sub_gnss-data_check.vi"("sel"=T3."GxGGA", "gnss str"=w15) -> ("val"=w13:bool, "TM"=w25:cluster{dbl, dbl})  [unwired: 6 in, 2 out]
    "GNGGA_val" <- w13
    n9 = case shown="참" "add str" {
      tunnel: w30 -> [w41 w44]
      tunnel: [w41 w43] -> w29
      tunnel: w15 -> [_ w42]
      frame False {
      }
      frame True {
        n10 = Concatenate Strings(w44, w42) -> (w43:string)
      }
    }
    "연결된 문자열" <- w29
    n11 = case shown="참" w13 {
      tunnel: w12 -> [w32 w36]
      tunnel: [w32 w35] -> w24
      tunnel: w25 -> [_ w34]
      frame False {
      }
      frame True {
        n12 = case shown="참" "graph arr" {
          tunnel: w36 -> [w37 w40]
          tunnel: [w37 w39] -> w35
          tunnel: w34 -> [_ w38]
          frame False {
          }
          frame True {
            n13 = Build Array (concatenate)(w40, w38) -> (w39:cluster{dbl, dbl}[])
          }
        }
        "LatLong" <- w34
      }
    }
    n14 = Wait (ms)(milliseconds to wait=u32 10 ("대기 시간 (ms)")) -> ()  [unwired: 1 out]
    n15 = Or(x="정지", y=w20) -> (x .or. y?=w18:bool)
    "XY 그래프" <- w12
    "n" <- w21
  }
  n16 = call "fgv_232_F9P.vi"("cmd"=enum16{"init", "read", "write", "close"}."close", "error in"=w3) -> ("error out"=w2:errorcluster)  [unwired: 7 in, 2 out]
  n17 = flat-sequence {
    tunnel: w2 -> [_]
    frame #0 {
    }
  }
